vi "Text control 2 v5.4.vi"() -> ()   [LabVIEW 2016]
panel:
  in  "Tab Control":enum32{"Main", "Other parameters"}(tab)
  out "Line running":i32
  out "Total lines":i32
  out "Path":path=path "C:/users/rlp38/09Apr2009LTtesting/test2.txt"
  out "I vs Vg":cluster{"Y data in":dbl[], "X data in":dbl[]}[](graph)
  out "Is max":dbl format="%.2e"
  out "Id max":dbl format="%.2e"
  out "Ig max":dbl format="%.2e"
  out "Imax vs time":cluster{"Y data in":dbl[], "X data in":dbl[]}[](graph)
  out "Imin vs time":cluster{"Y data in":dbl[], "X data in":dbl[]}[](graph)
  out "I vs Vd":cluster{"Y data in":dbl[], "X data in":dbl[]}[](graph)
  in  "Script":string="#pulsedstressV d 0.03 20 0 0.5 0.0827 5\n#\n#itime m\n#gaterangemode a\n#drainrangemode a\n#pulsed on 0.05 0 0.02\n#transfer d -10 40 1 5 40 35\n#transfer d -10 40 1 5 40 35\n#transfer d -10 40 1 5 40 35\n#output d 0 40 20 0 40 1\n#\n#\n#sample 1 0.008 221 6 0.003\n#samplei 400e-6 200 6 0.002 0.1\n#vsu2pulse -10 4\n#\n#stressV 0.016 0.03 2e-4 0.1e-3 11\n#stressI 220e-7 0.08 15\n#transfer s -1 1 0.5 -0.005 0.005 0.005\n#output s 0 0 0 -0.008 0.008 0.002"
  out "Command running:":string
  out "Serial port data":string
  out "Elapsed Time":dbl caption="Elapsed Time (s)"
  in  "Units":u16(ring)=1 items=["Seconds", "Minutes", "Hours"]
  in  "Time Offset":dbl caption="Set Start Time (s)"
  in  "Reset":bool
  in  "Auto Reset":bool
  in  "integration time":u32(slide) max=2 step=1 scale=0.0..2.0
  in  "Interrupt run":bool
  out "Is on":dbl format="%.2e"
  out "Id on":dbl format="%.2e"
  out "Ig on":dbl format="%.2e"
  out "Ion vs time":cluster{"Y data in":dbl[], "X data in":dbl[]}[](graph)
  out "Ioff vs time":cluster{"Y data in":dbl[], "X data in":dbl[]}[](graph)
  out "Ig min":dbl format="%.2e"
  out "Id min":dbl format="%.2e"
  out "Is min":dbl format="%.2e"
  out "Is off":dbl format="%.2e"
  out "Id off":dbl format="%.2e"
  out "Ig off":dbl format="%.2e"
  in  "Step delay /s":dbl format="%.2f"
  in  "Integration time (long)":dbl=0.32 min=0.04 max=2.0 step=0.02 format="%.2f"
  in  "Integration time (short)":dbl=0.0019 min=8e-05 max=0.0019 step=8e-05 format="%^.0e"
  in  "delay time /s":dbl format="%.2f"
  in  "hold time /s":dbl format="%.2f"
  in  "Gate: Compliance":dbl=0.001 format="%.8f"
  in  "Drain: Compliance":dbl=0.001 format="%.8f"
  in  "Source/Drain Range":u8(slide)=6 max=11 scale=0.0..11.0
  in  "Source/Drain\nRange mode":u16(ring) items=["Auto", "Limited", "Fixed"]
  in  "Gate Range":u8(slide)=6 max=11 scale=0.0..11.0
  in  "Gate Range\nmode":u16(ring) items=["Auto", "Limited", "Fixed"]
  in  "Panel Controls":T1={"Emergency Stop"=refnum, "TransGraph Max"=1e-05, "Text/Graph (text=false)"=TRUE} {"TransGraph Max" format="%.2e"}
  in  "Panel Controls 2":T2={"Emergency Stop"=refnum, "TransGraph Max"=1e-05, "Text/Graph (text=false)"=TRUE, "TransGraph Min"=1e-11} {"TransGraph Min" format="%.2e"; "TransGraph Max" format="%.2e"}
  in  "SMU4":cluster{"on/off":bool, "Voltage":dbl} {"Voltage" min=-100.0 max=100.0 format="%.2f"}
  in  "Full Reset":bool
  in  "Standby":T3
  out "error out":errorcluster
  in  "Delay before read (ms)":u32=1000
  in  "byte count":u32=64
  in  "Serial End Mode for Reads":u16(ring)=2 items=["None", "LastBit", "TermChar"]
  in  "Timeout (ms)":u32=10000
  in  "Enable Termination\nChar (T)":bool=TRUE
  in  "Termination char\n(0xA = '\\n' = LF)\n(0xD = '\\r' = CR)":u8=13 format="%.0x"
  in  "flow control":u16(ring) items=["None"=0, "XON/XOFF"=1, "RTS/CTS"=2, "DTR/DSR"=4]
  in  "stop bits":u16(ring)=10 items=["1.0"=10, "1.5"=15, "2.0"=20]
  in  "parity":u16(ring) items=["None", "Odd", "Even", "Mark", "Space"]
  in  "data bits":u16=8 min=5 max=8 step=1
  in  "VISA resource name":refnum<visa-resource-name>="COM6"
  in  "baud rate":u32=9600
  in  "Gate":T4={"Gate Start"=0.0, "Gate Stop"=2.0, "Gate Step (linear only)"=1.0, "Gate Compliance"=0.0001, "Gate PComp"=0.0, "Range mode"=0, "Range"=6} {"Range" max=11 scale=0.0..11.0; "Range mode" items=["Auto", "Limited", "Fixed"]; "Gate PComp" format="%^.2e"; "Gate Compliance" format="%^.2e"; "Gate Step (linear only)" format="%^.4e"; "Gate Stop" format="%^.4e"; "Gate Start" format="%^.4e"}
  in  "Drain 2":T5={"Drain Start"=0.0, "Drain Stop"=2.0, "Drain Compliance"=0.0001, "Drain Step"=1.0, "Drain PComp"=0.0, "Range mode"=0, "Range"=6} {"Range" max=11 scale=0.0..11.0; "Range mode" items=["Auto", "Limited", "Fixed"]; "Drain PComp" format="%^.2e"; "Drain Step" format="%^.4e"; "Drain Compliance" format="%^.2e"; "Drain Stop" format="%^.4e"; "Drain Start" format="%^.4e"}
  in  "Timings 2":T6={"integration time"=0, "Short/Long integration time"=0.00064, "hold time (sec)"=0.0, "delay time (sec)"=0.0, "Step Time (0 disables)"=0.0, "sweep method"=0, "Pulse period"=0.005, "Base voltage"=0.0, "Pulse width"=0.0005} {"Pulse width" min=0.0005 max=0.1 step=0.0001 format="%.4f"; "Base voltage" format="%^.4e"; "Pulse period" min=0.005 max=1.0 step=0.0001 format="%.4f"; "sweep method" items=["Continuous", "Pulsed"]; "Step Time (0 disables)" format="%.2f"; "delay time (sec)" format="%.4f"; "hold time (sec)" format="%.4f"; "Short/Long integration time" format="%^.0e"; "integration time" scale=0.0..2.0}
  # "Time"
  # "1\n2\n3\n4\n5\n6\n7\n8\n9\n10\n11\n12\n13\n14\n15\n16\n17\n18\n19\n20"
  # "Syntax:\nitime [s|m|l]\ngaterangemode [a|l|f]\ndrainrangemode [a|l|f]\npulsed [on|off] PulsePeriod(sec) PulseBaseVoltage PulseONWidth(sec)\nstandby [on l off]\nwait NumMilliseconds\nwait-min NumMinutes\n# texthere = comment\ntransfer [s|d] VgStart VgStop VgStep VdStart VdStop VdStep\noutput [s|d] VgStart VgStop VgStep VdStart VdStop VdStep\nsample Vg Vd NumSamples Time(s) SampleInterval(s)\nsamplei Idg NumSamples Time(s) SampleInterval(s) VDGcompliance\n100 samples is approximately 13 seconds with medium integration\n# if in doubt use SampleInterval(s) = 0.004\nstressV VG VD IGcompliance IDcompliance Duration(sec)\nstressI IDG VDGcompliance Duration(sec)\nvsu2pulse Bias Duration(s)\npulsedstressV [s|d] VEstop VgON VgOFF Period(s) PulseONwidth(s) Vd\nsample-fpp Vg Vd NumSamples Time\nresample-fpp Vg Vd\ntransfer-fpp [s|d] VgStart VgStop VgStep VdStart VdStop VdStep\noutput-fpp [s|d] VgStart VgStop VgStep VdStart VdStop VdStep\nserial SerialPortCommand"
  # "Serial port settings"
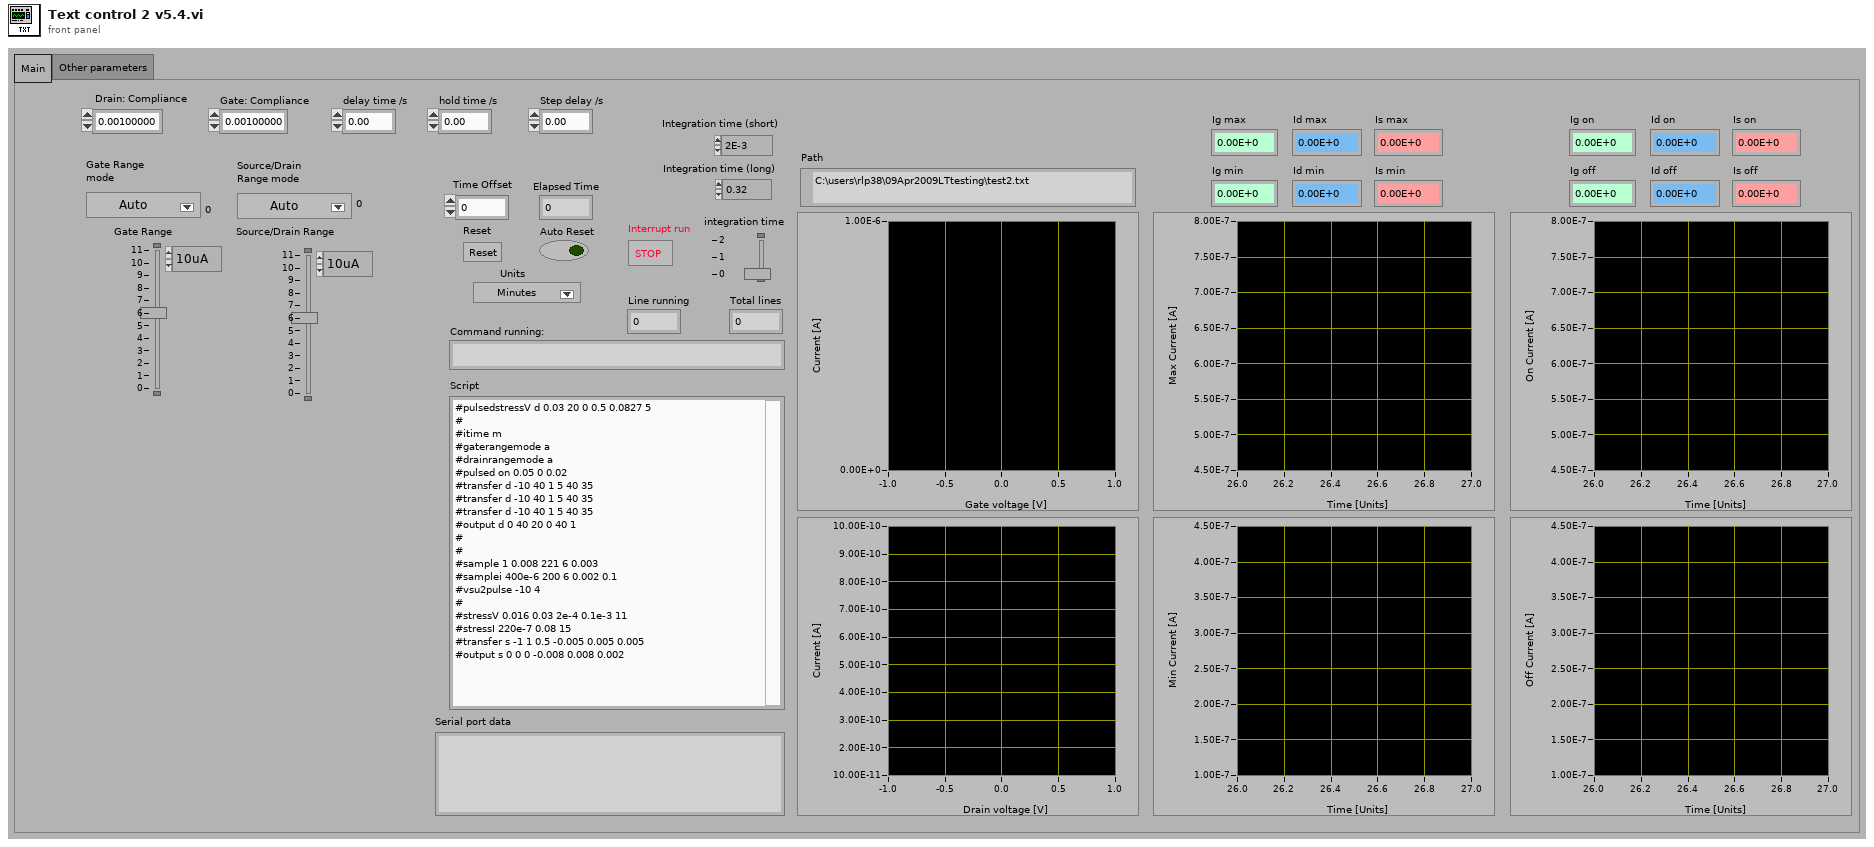
[diagram p1: front panel]
types:
  T1 = cluster{"Emergency Stop":refnum<vi>, "TransGraph Max":dbl, "Text/Graph (text=false)":bool}
  T2 = cluster{"Emergency Stop":refnum<vi>, "TransGraph Max":dbl, "Text/Graph (text=false)":bool, "TransGraph Min":dbl}
  T3 = cluster{"Gate Standby":bool, "Drain Standby":bool}
  T4 = cluster{"Gate Start":dbl, "Gate Stop":dbl, "Gate Step (linear only)":dbl, "Gate Compliance":dbl, "Gate PComp":dbl, "Range mode":u16, "Range":u8}
  T5 = cluster{"Drain Start":dbl, "Drain Stop":dbl, "Drain Compliance":dbl, "Drain Step":dbl, "Drain PComp":dbl, "Range mode":u16, "Range":u8}
  T6 = cluster{"integration time":u32, "Short/Long integration time":dbl, "hold time (sec)":dbl, "delay time (sec)":dbl, "Step Time (0 disables)":dbl, "sweep method":u16, "Pulse period":dbl, "Base voltage":dbl, "Pulse width":dbl}
  T7 = enum16{"open", "replace", "create", "open or create", "replace or create", "replace or create with confirmation"}
  T8 = cluster{"V2 Start":dbl, "V2 Step":dbl, "Number of points":i32}
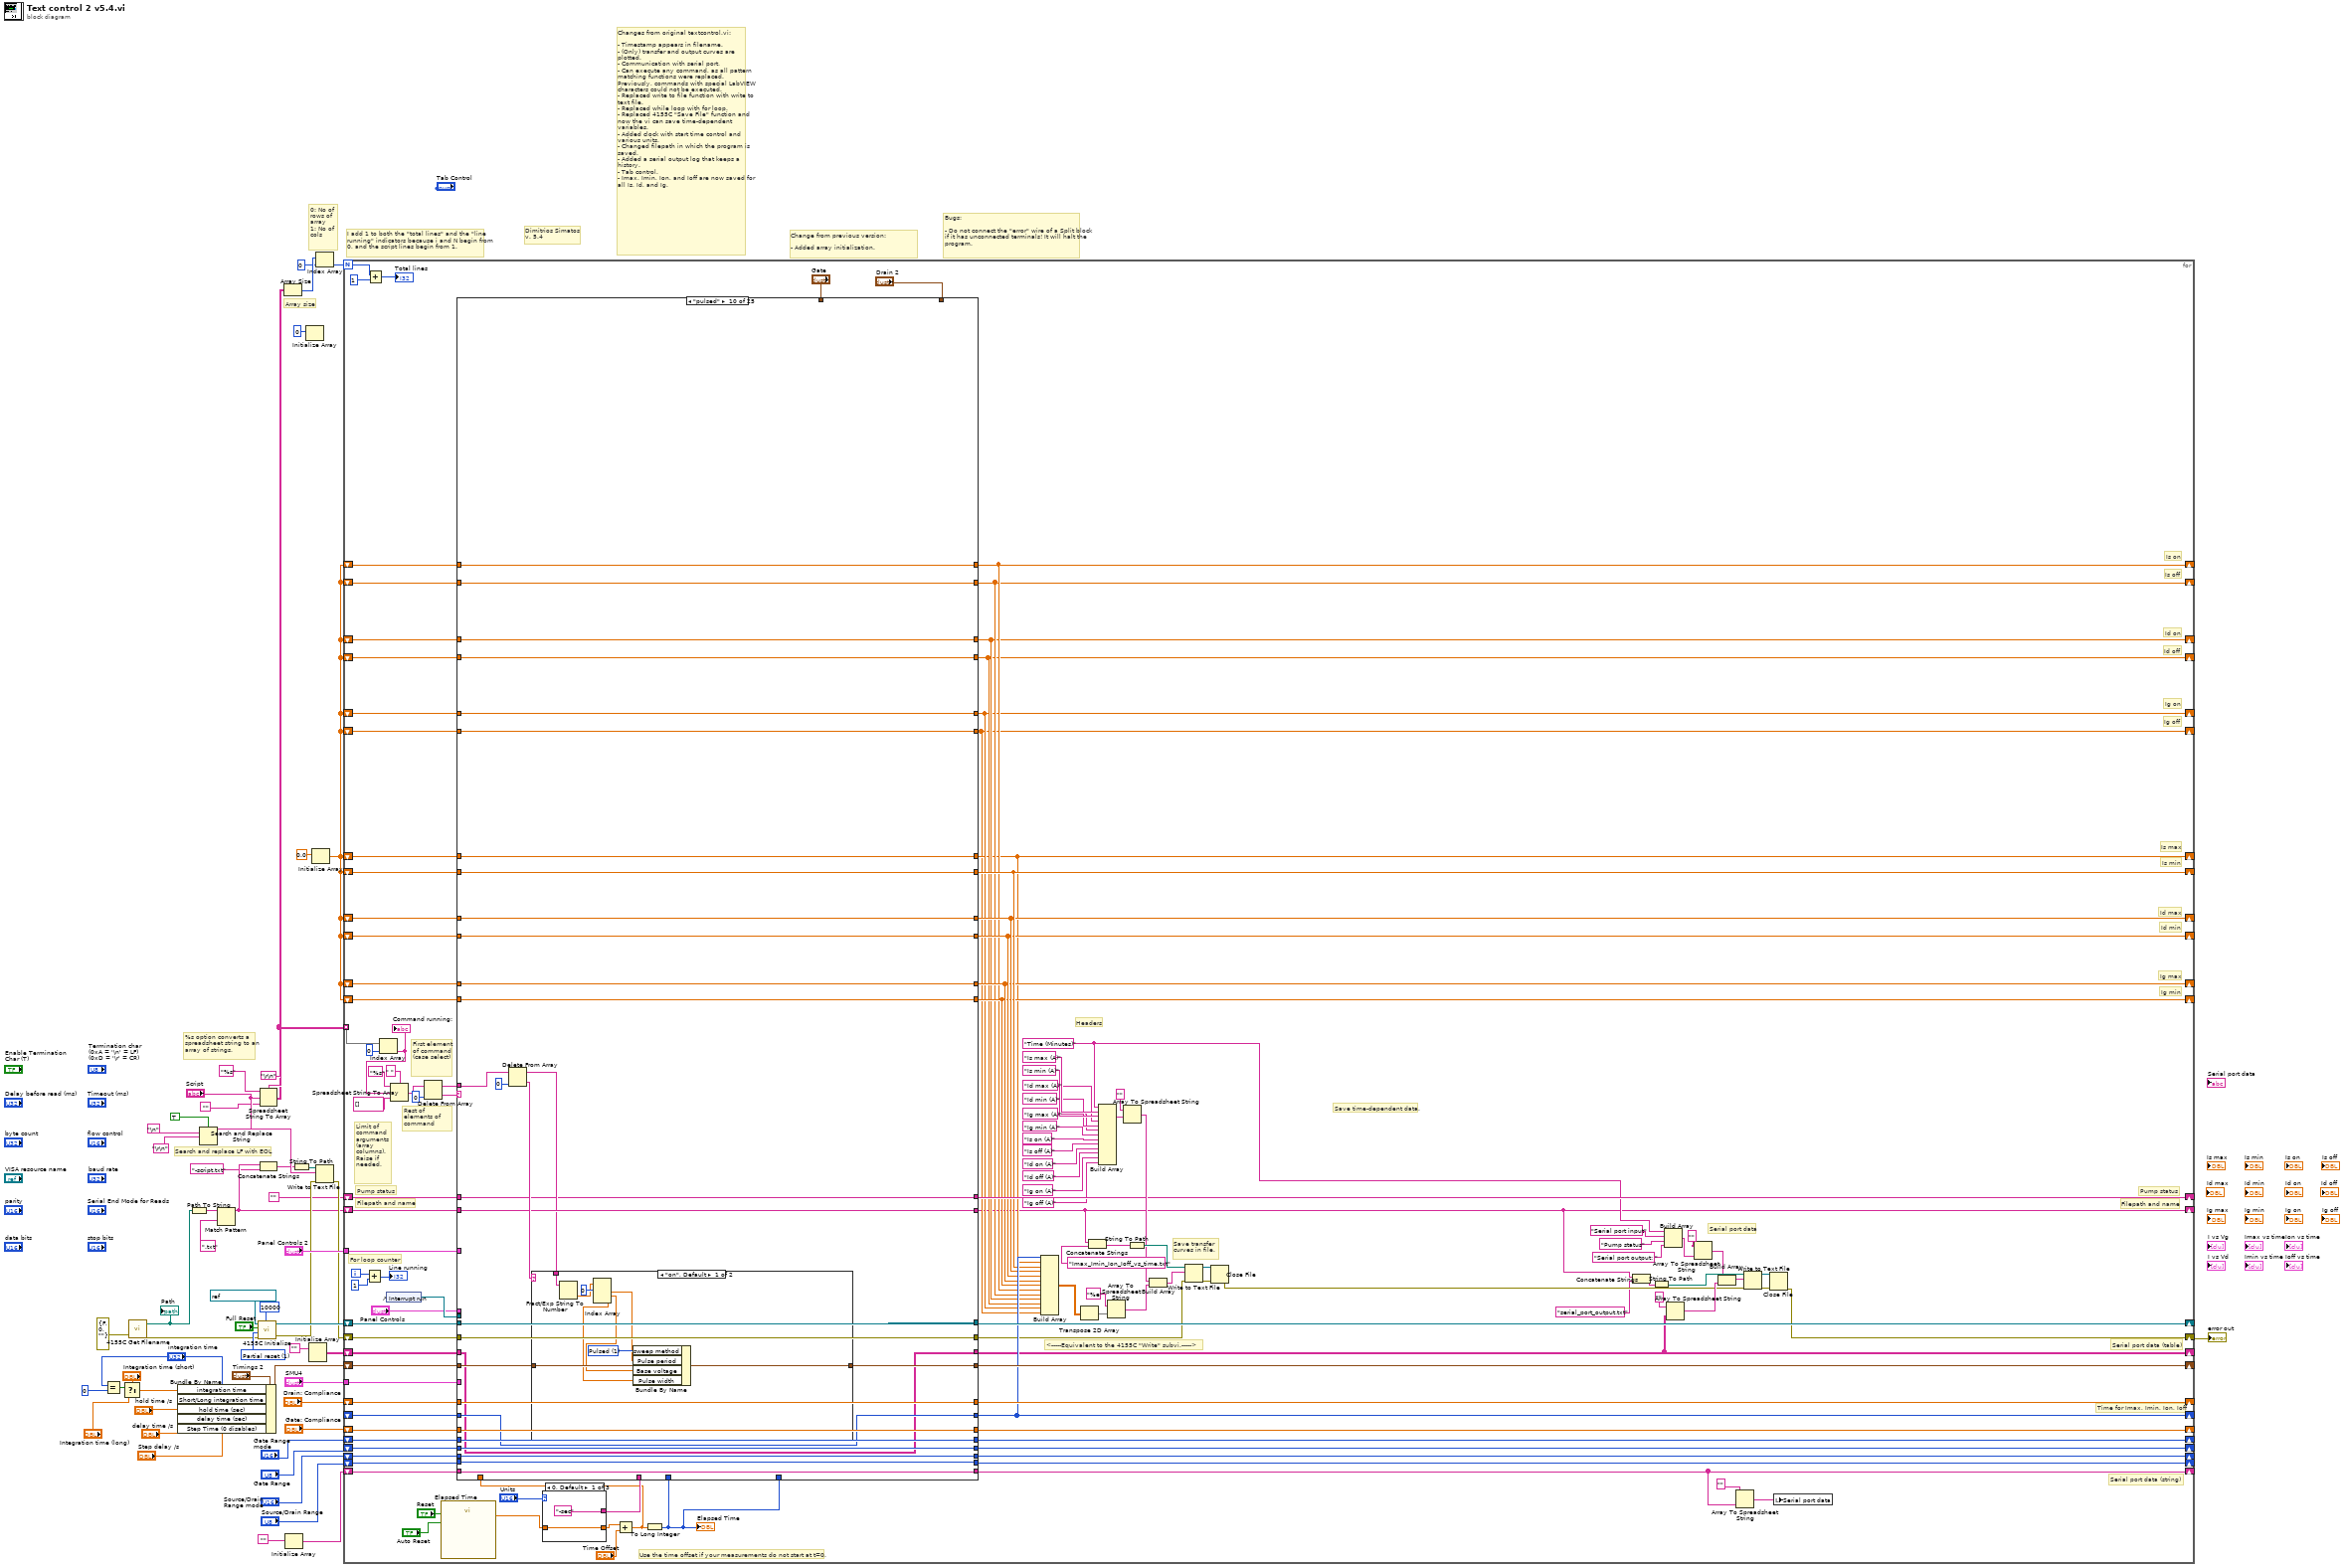
[diagram p0: block diagram]
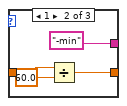
[diagram p2: hidden frame]
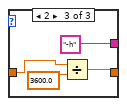
[diagram p3: hidden frame]
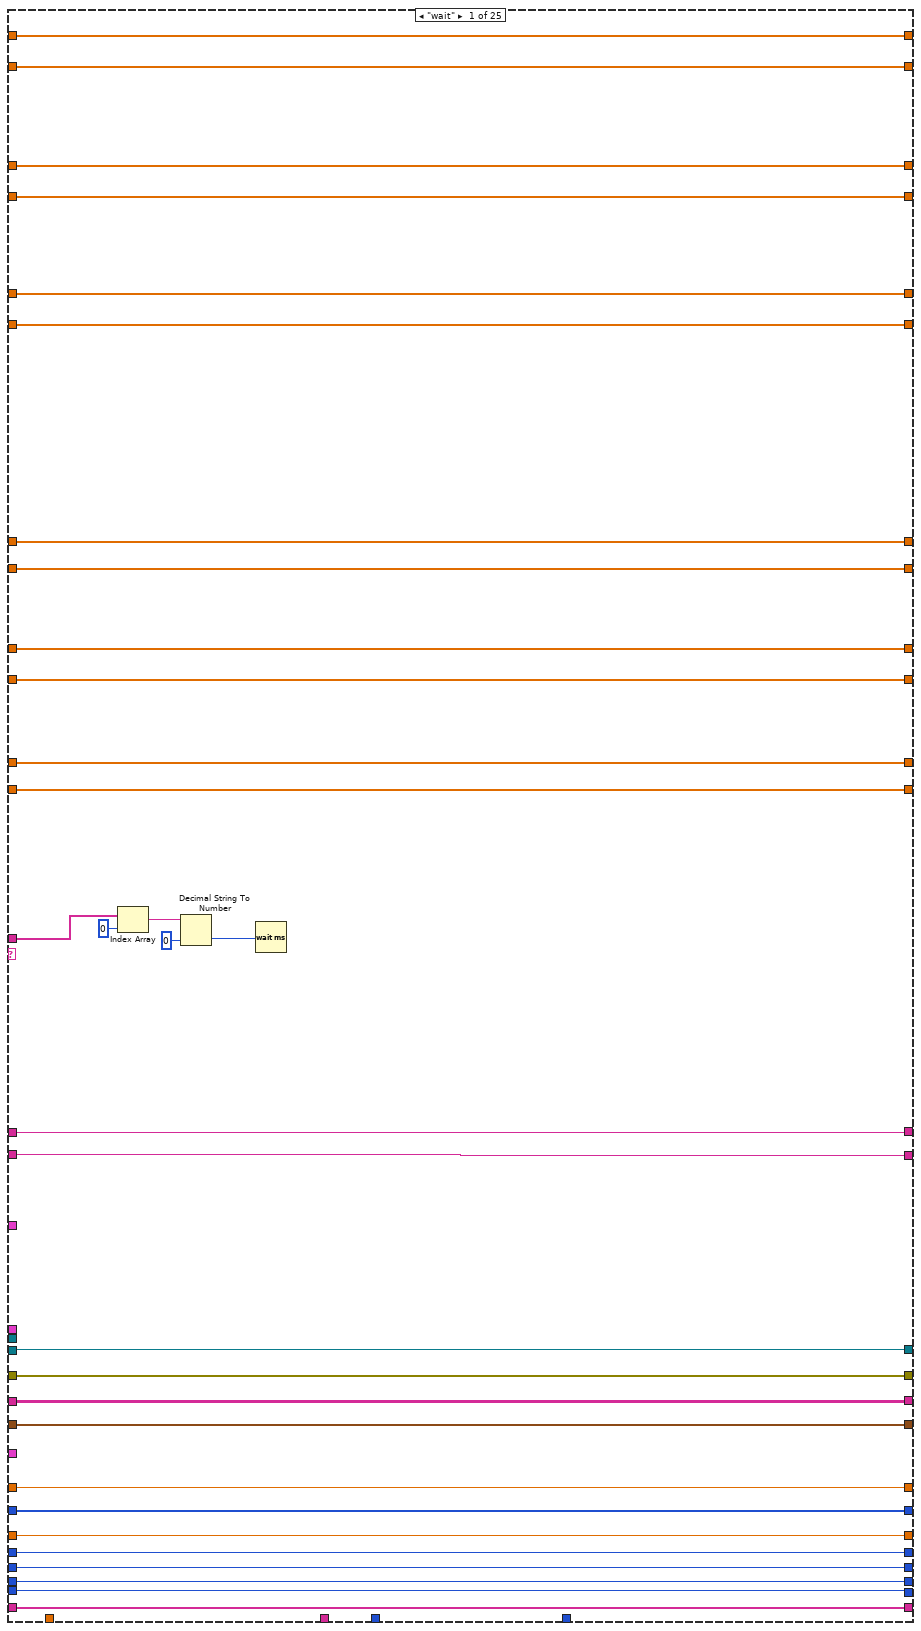
[diagram p4: hidden frame]
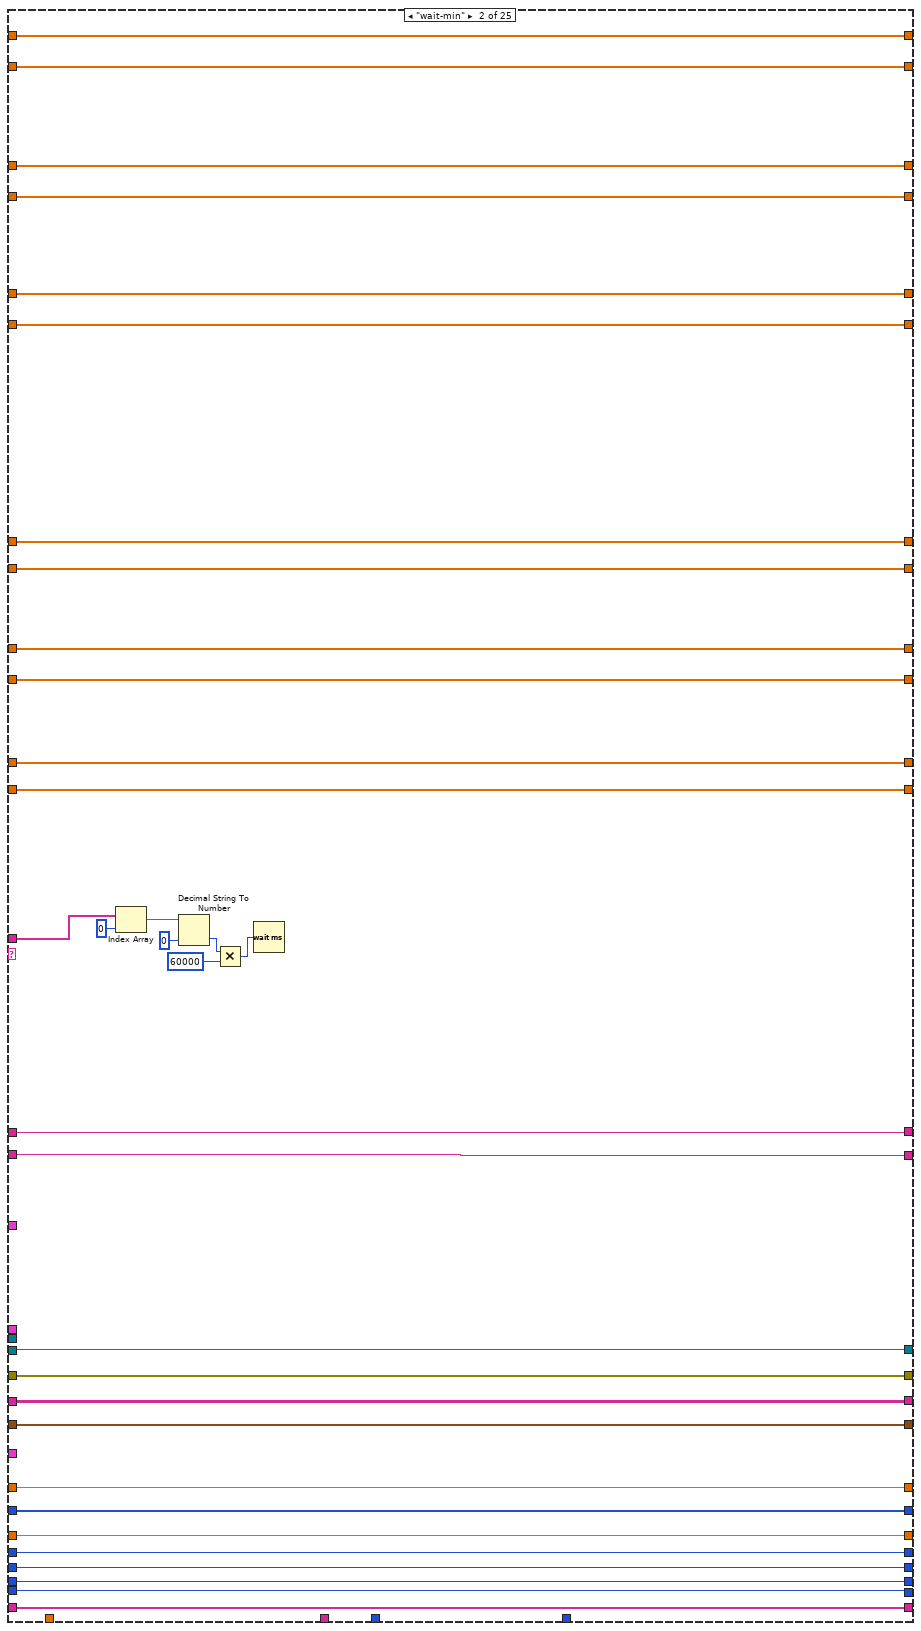
[diagram p5: hidden frame]
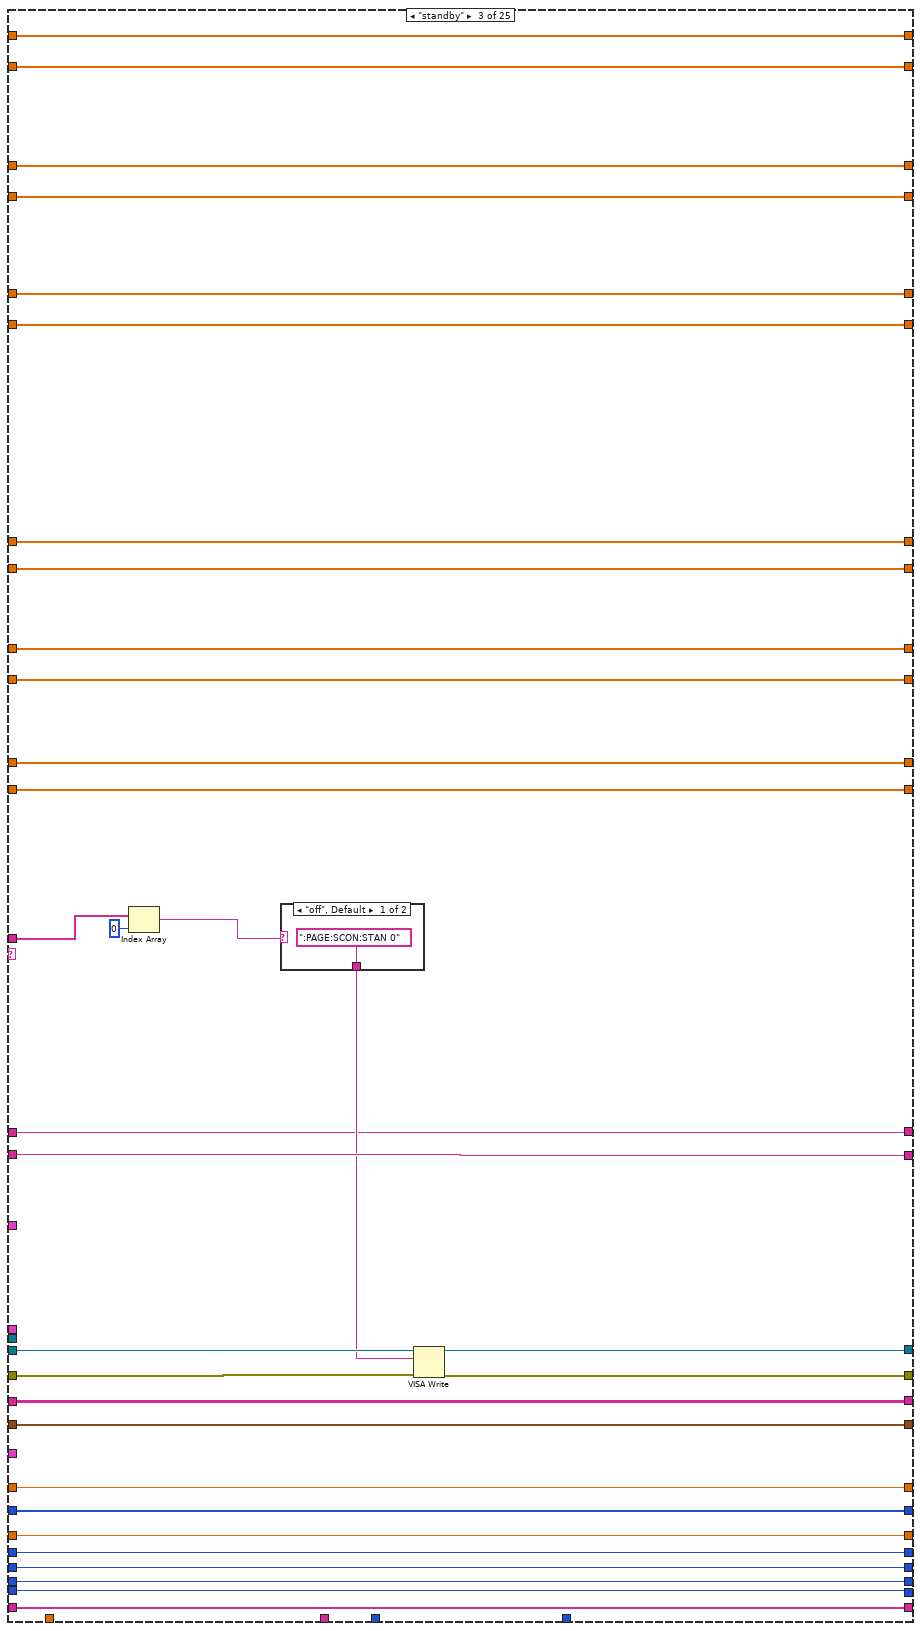
[diagram p6: hidden frame]
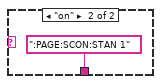
[diagram p7: hidden frame]
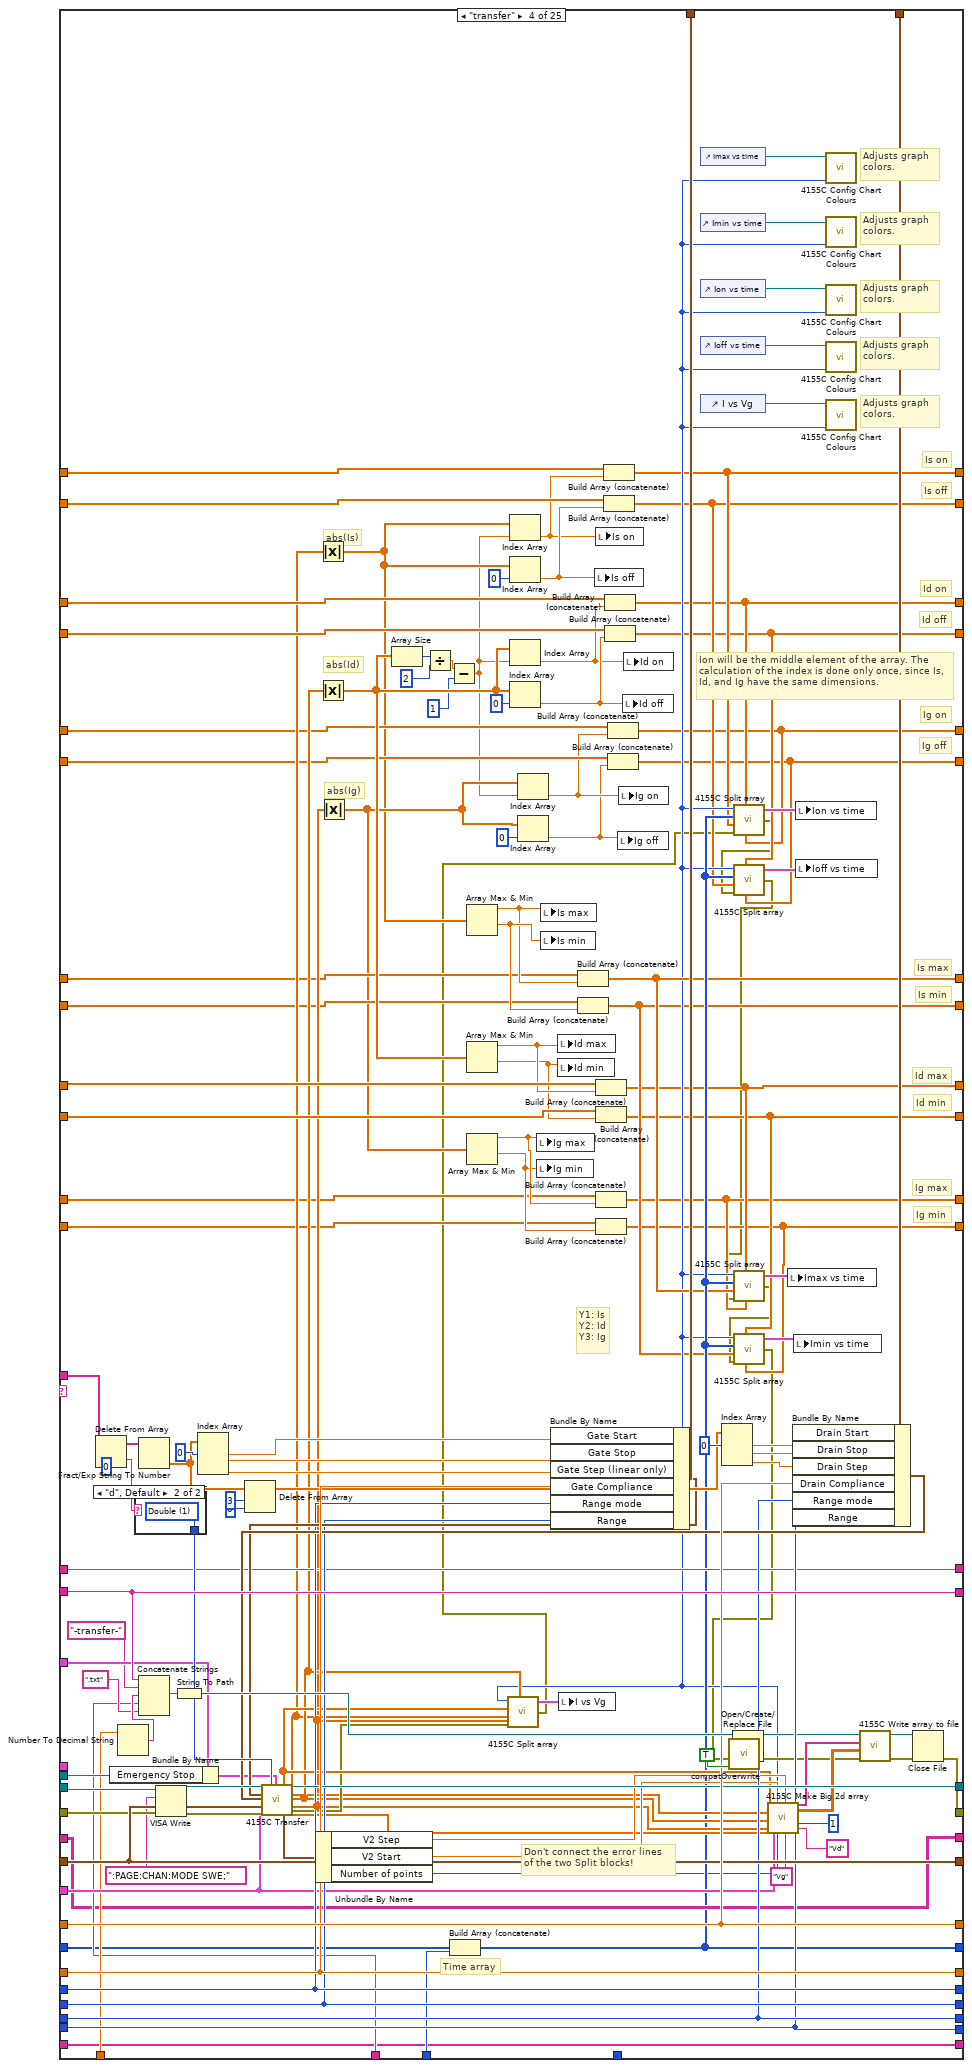
[diagram p8: hidden frame]
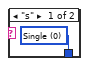
[diagram p9: hidden frame]
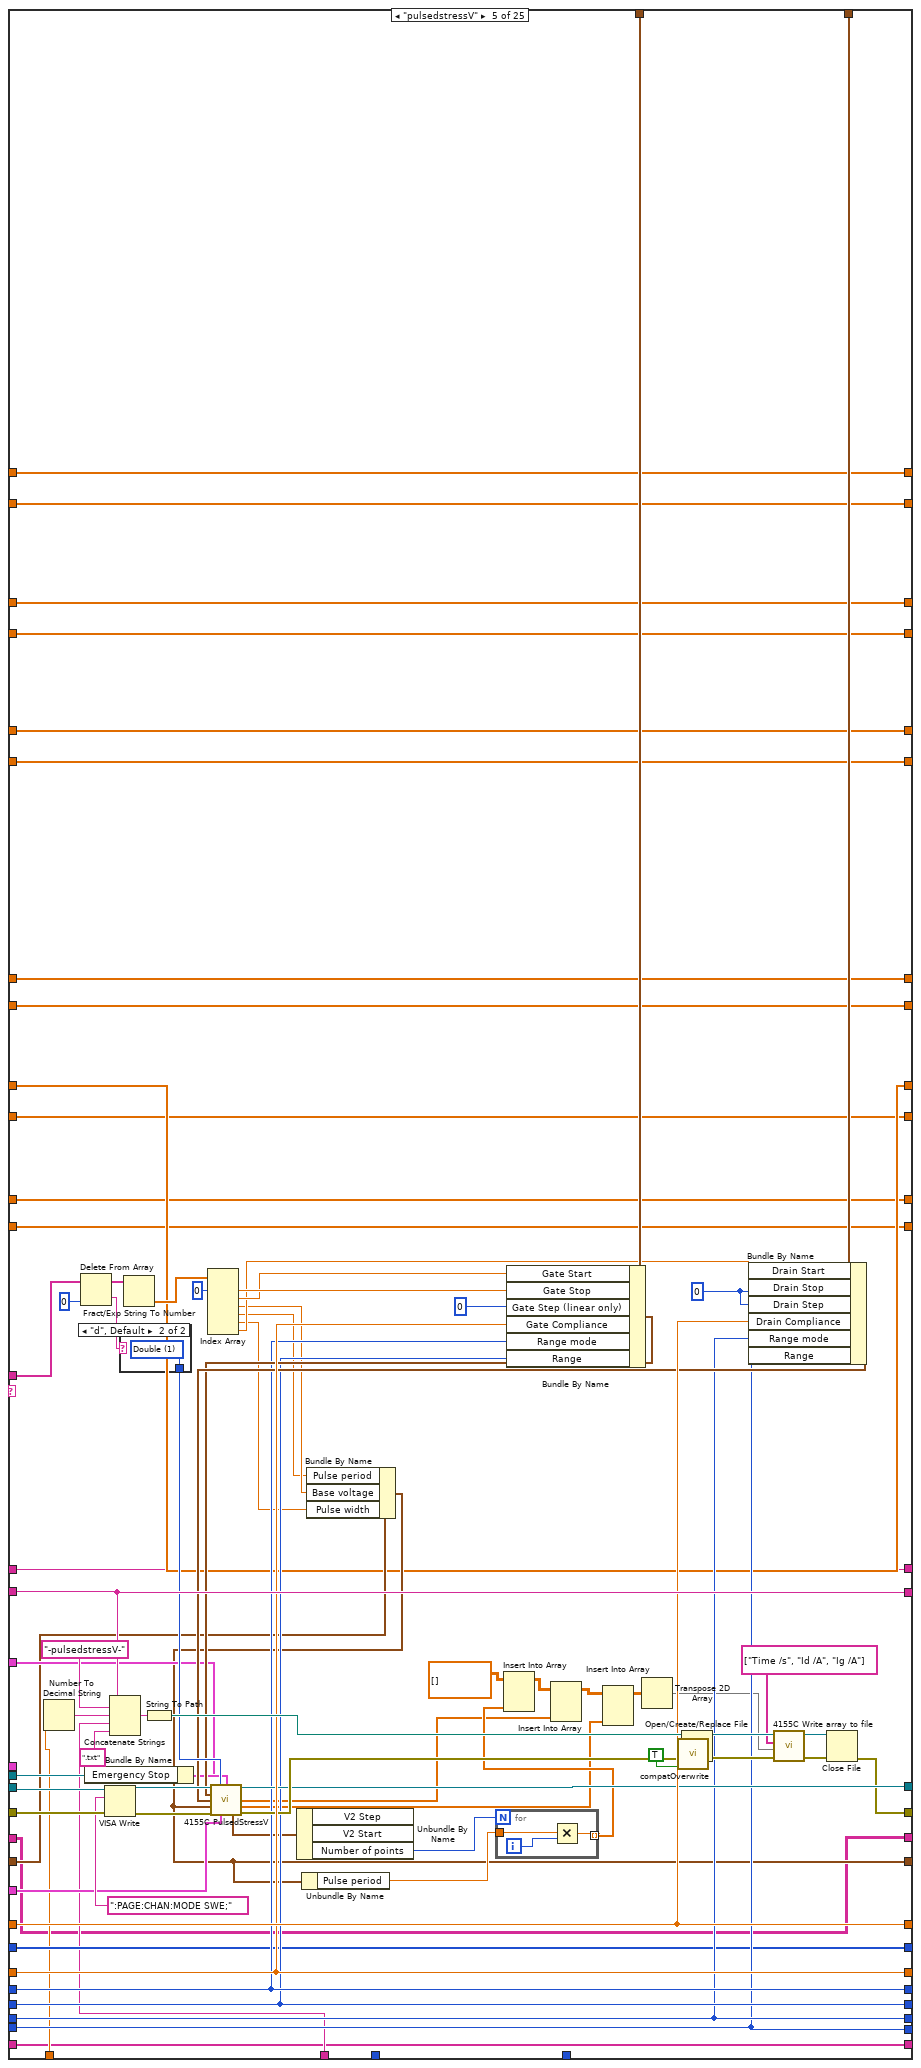
[diagram p10: hidden frame]
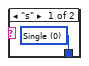
[diagram p11: hidden frame]
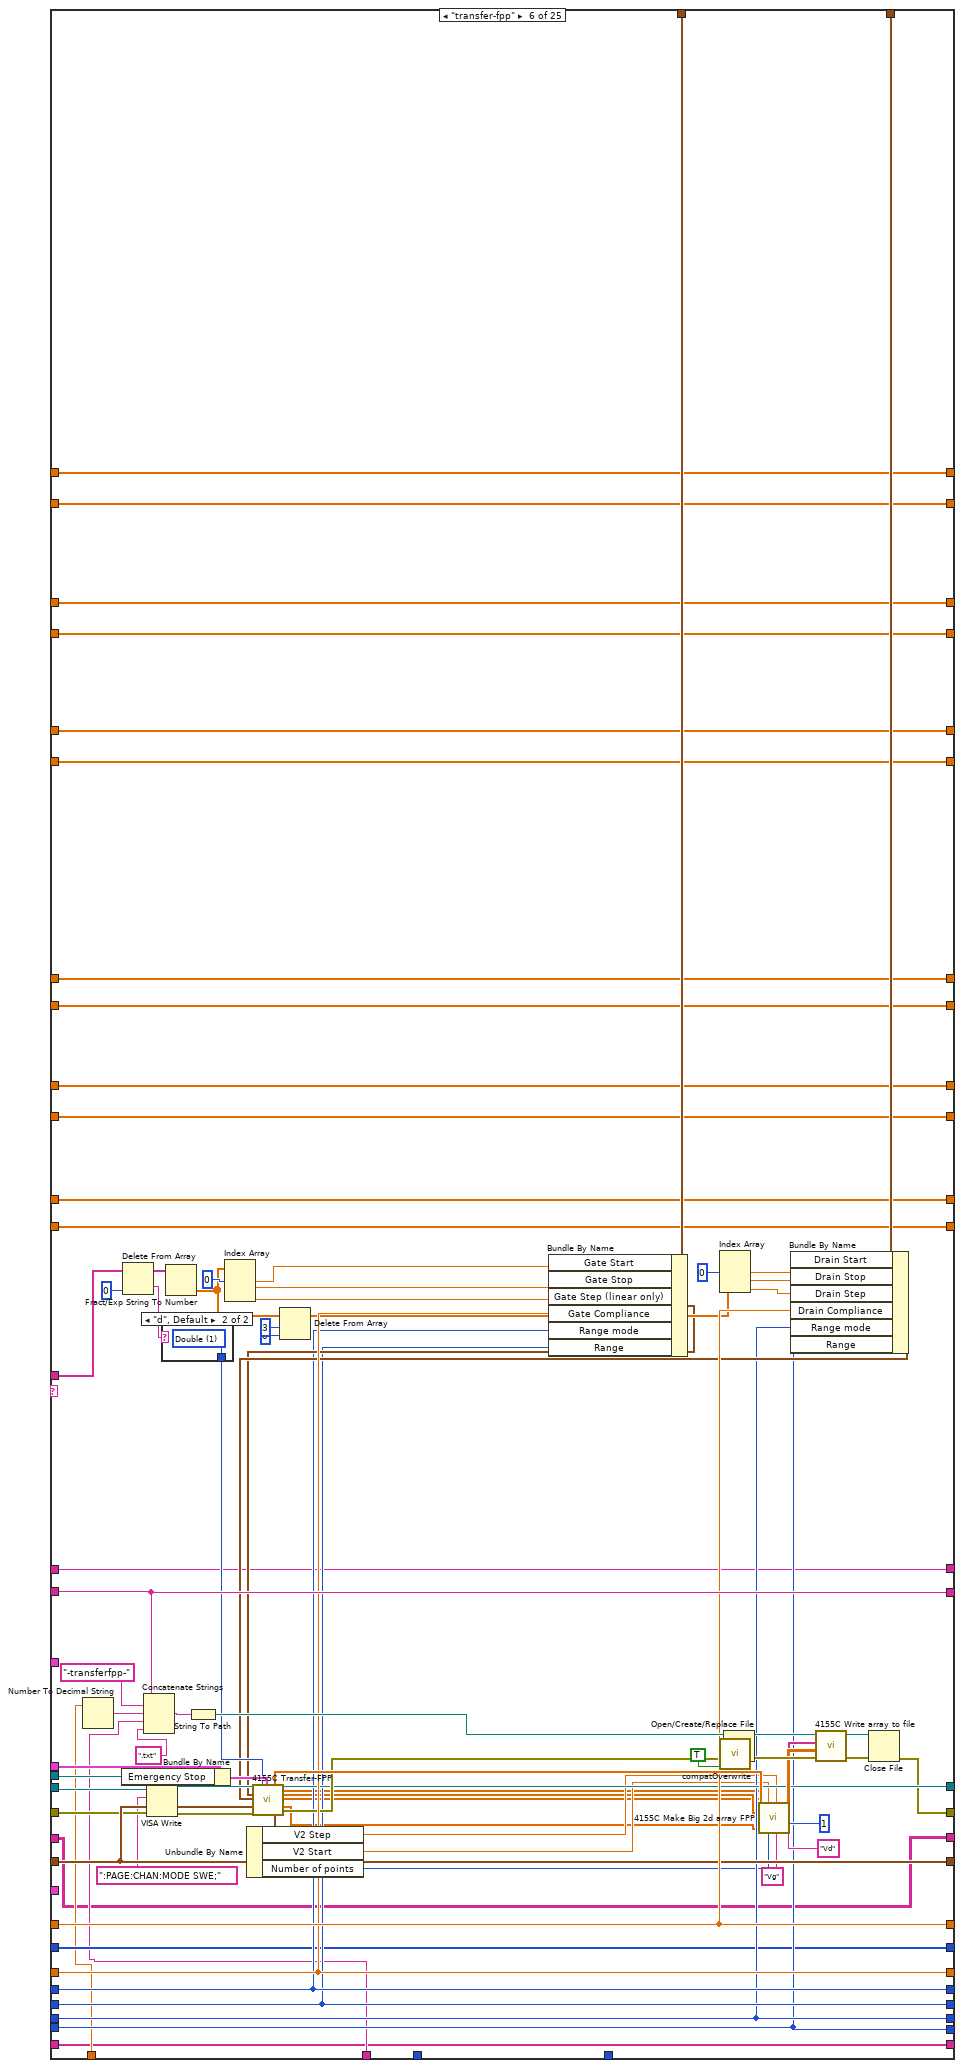
[diagram p12: hidden frame]
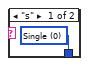
[diagram p13: hidden frame]
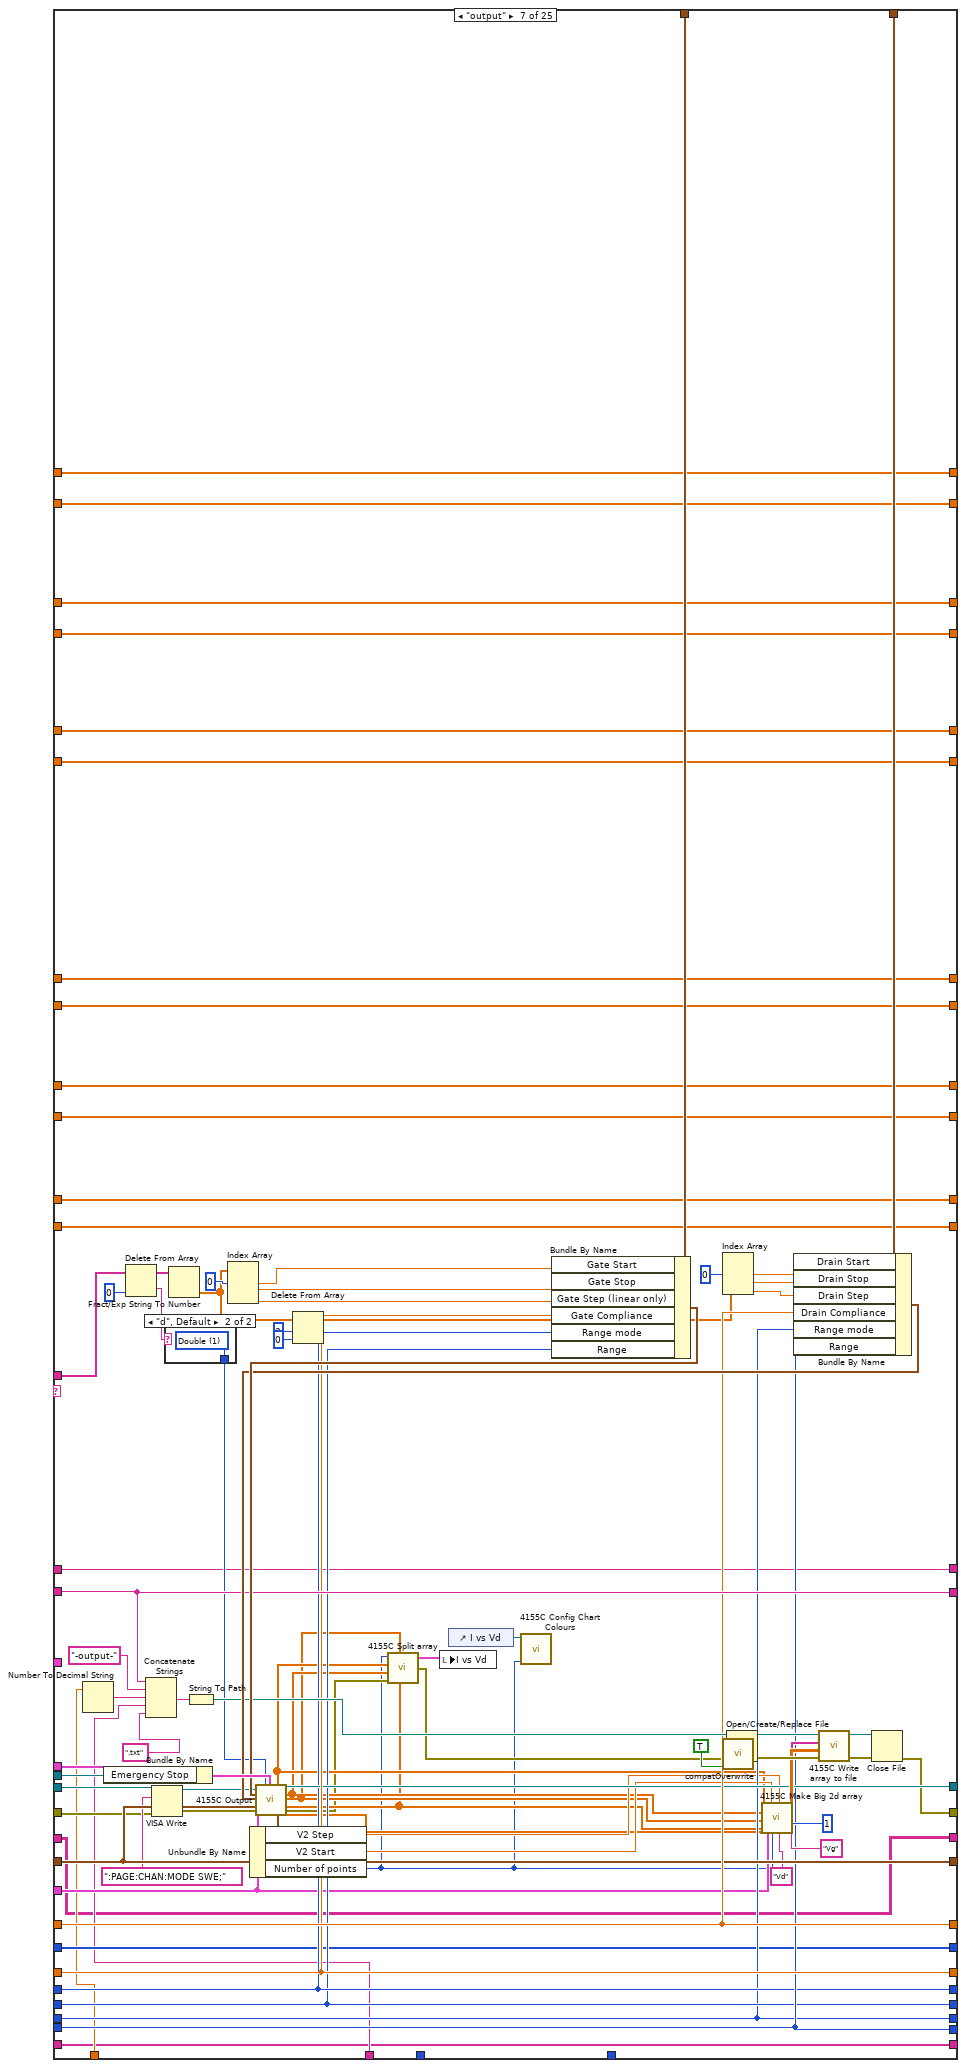
[diagram p14: hidden frame]
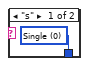
[diagram p15: hidden frame]
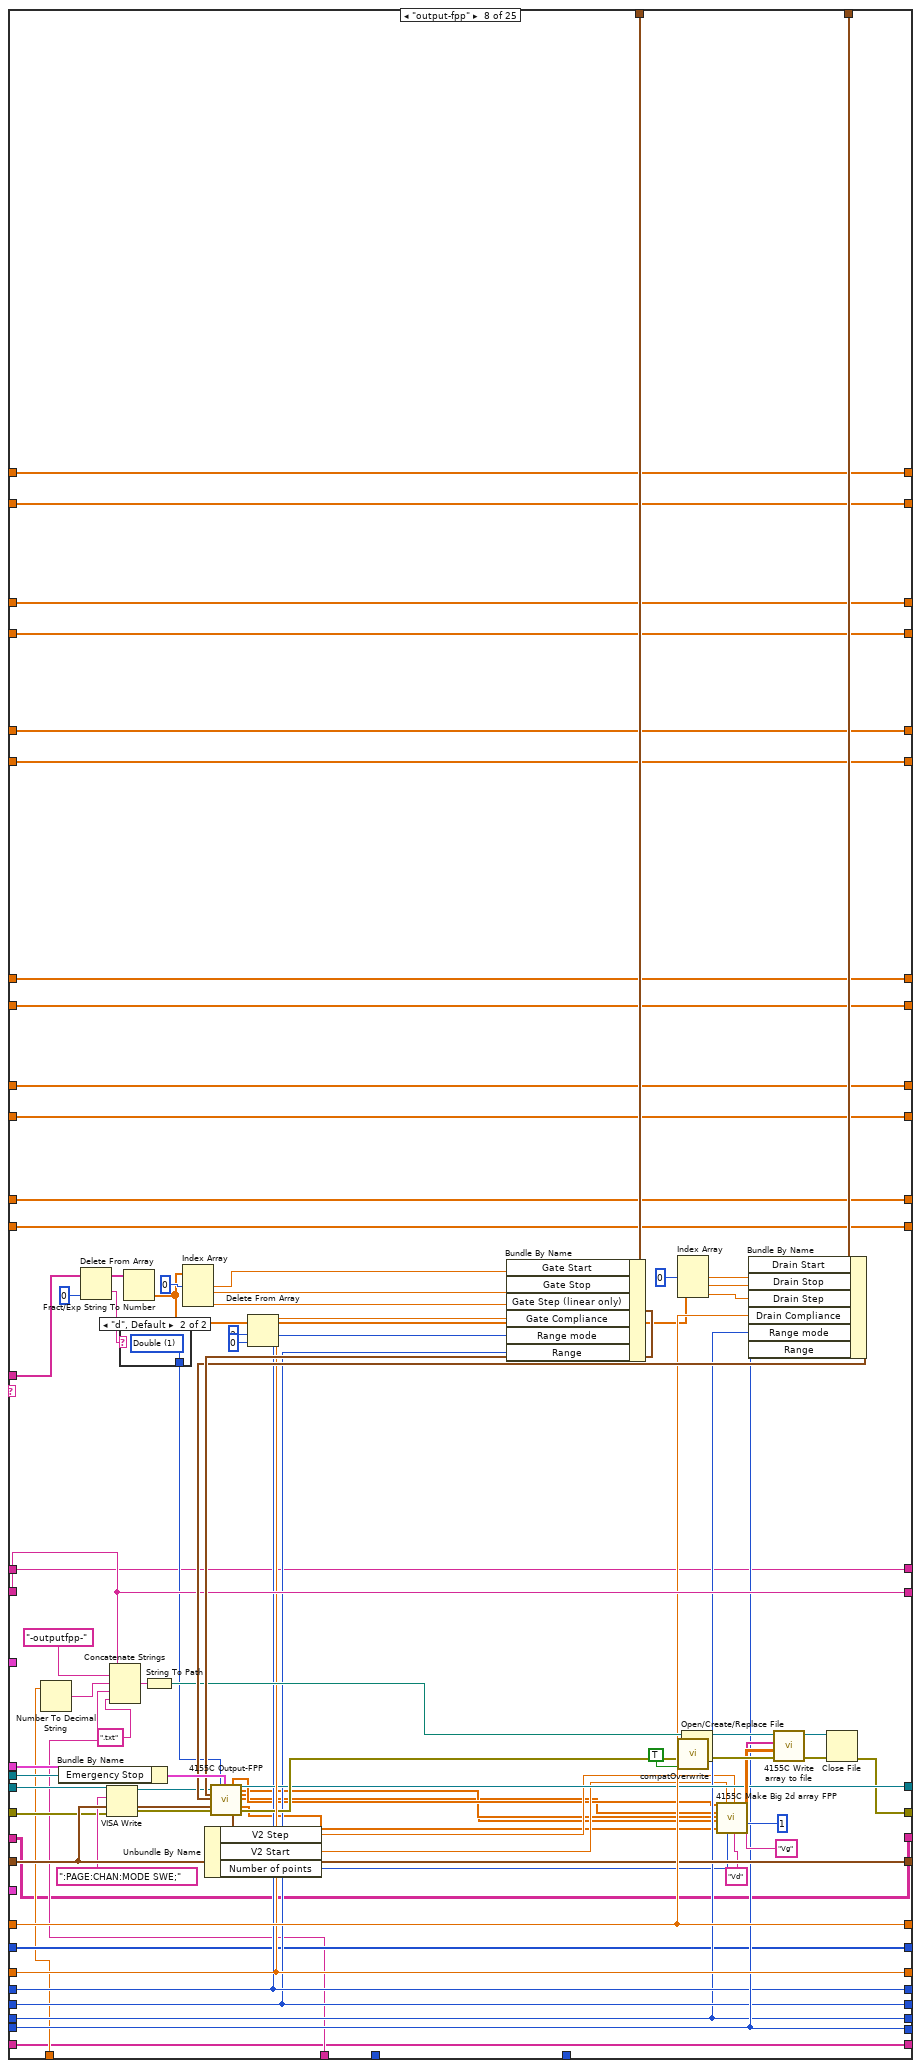
[diagram p16: hidden frame]
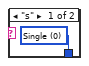
[diagram p17: hidden frame]
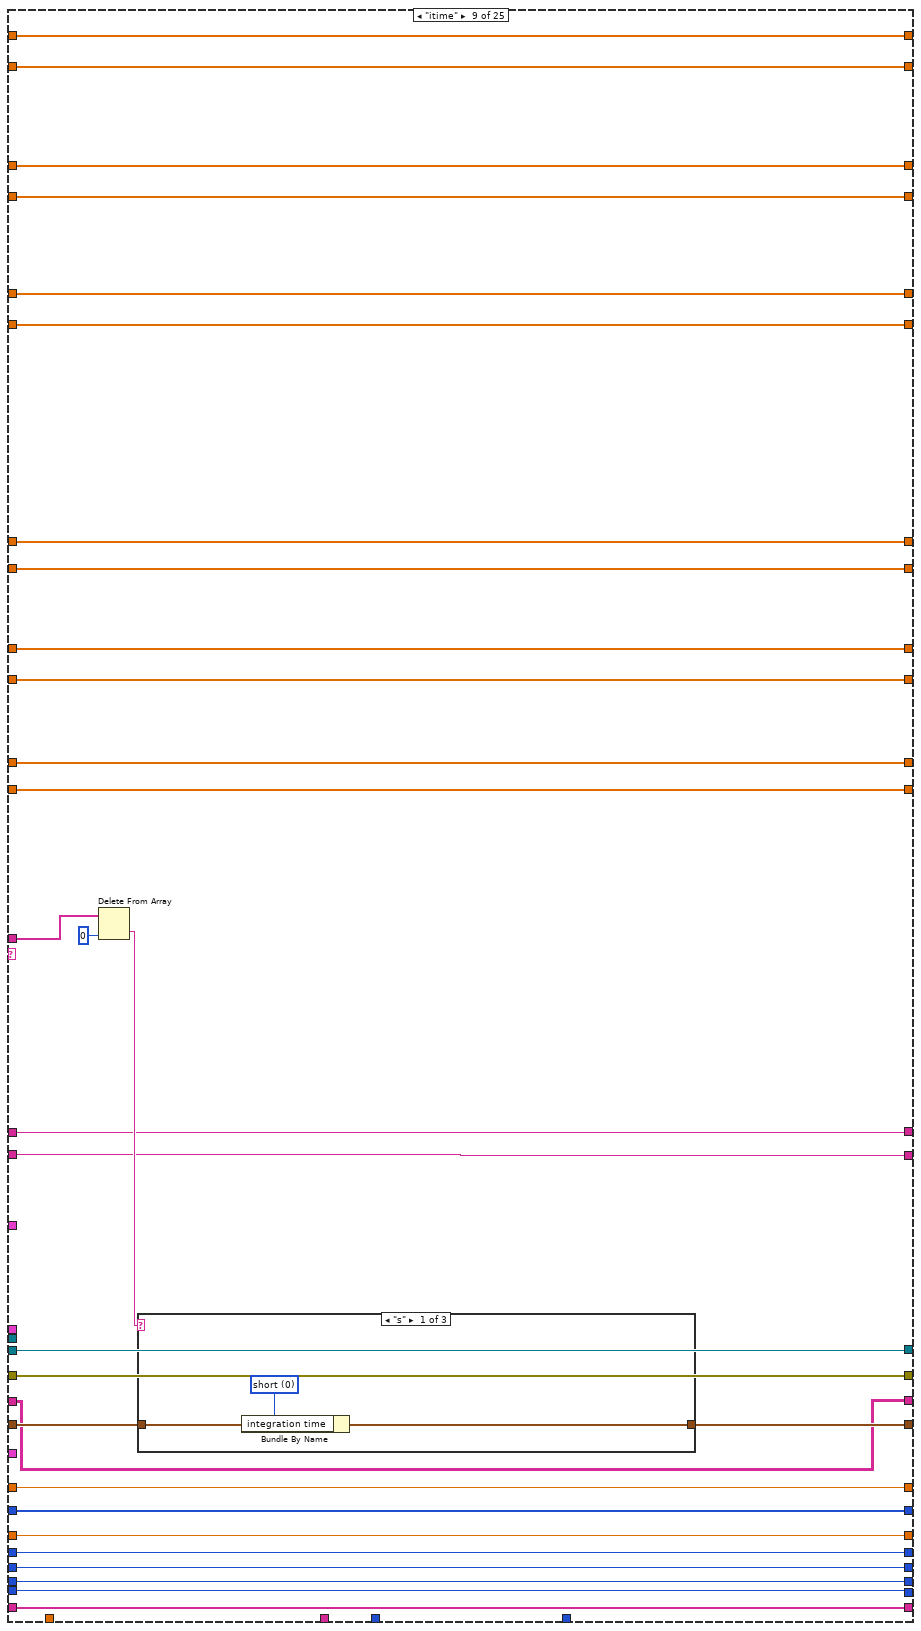
[diagram p18: hidden frame]
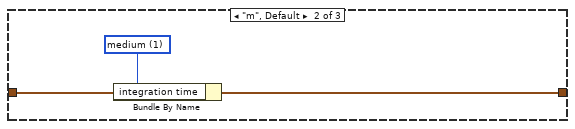
[diagram p19: hidden frame]
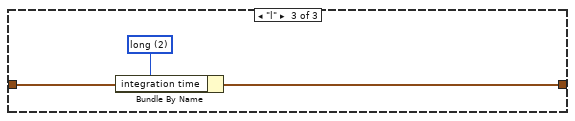
[diagram p20: hidden frame]
diagram:
  w47 = u16 1 items=["Reset All", "Partial reset"] ("Type of reset")
  # "Change from previous version:\n\n- Added array initialization."
  # "I add 1 to both the \"total lines\" and the \"line running\" indicators because i and N begin from 0, and the script lines begin from 1."
  # "Bugs:\n\n- Do not connect the \"error\" wire of a Split block if it has unconnected terminals! It will halt the program."
  # "Array size"
  # "%s option converts a spreadsheet string to an array of strings."
  # "0: No of rows of array\n1: No of cols"
  # "Dimitrios Simatos\nv. 5.4"
  # "Changes from original textcontrol.vi:\n\n- Timestamp appears in filename.\n- (Only) transfer and output curves are plotted.\n- Communication with serial port.\n- Can execute any command, as all pattern matching functions were replaced. Previously, commands with special LabVIEW characters could not be executed.\n- Replaced write to file function with write to text file.\n- Replaced while loop with for loop.\n- Replaced 4155C \"Save File\" function and now the vi can save time-dependent variables.\n- Added clock with start time control and various units.\n- Changed filepath in which the program is saved.\n- Added a serial output log that keeps a history.\n- Tab control.\n- Imax, Imin, Ion, and Ioff are now saved for all Is, Id, and Ig."
  # "Search and replace LF with EOL"
  n1 = Equal?(x="integration time", y=u32 0) -> (x = y?=w51:bool)
  n2 = Select(t="Integration time (short)", s=w51, f="Integration time (long)") -> (s? t:f=w55:dbl)
  n3 = call "4155C Get Filename.vi"("error in (no error)"=errorcluster {"status"=FALSE, "code"=0, "source"=""}) -> ("error out"=w42:errorcluster, "path"=w17:path)  [unwired: 2 in, 1 out]
  "Path" <- w17
  n4 = Bundle By Name(cluster="Timings 2", "integration time"="integration time", "Short/Long integration time"=w55, "hold time (sec)"="hold time /s", "delay time (sec)"="delay time /s", "Step Time (0 disables)"="Step delay /s") -> (w40:T6)
  n5 = Path To String(path=w17) -> (string=w18:string)
  n6 = Search and Replace String(replace all?=TRUE ("replace all? (F)"), input string="Script", search string="\n", replace string="\r\n") -> (result string=w30:string)  [unwired: 4 in, 3 out]
  n7 = Match Pattern(string=w18, regular expression=".txt") -> (before substring=w2:string)  [unwired: 1 in, 3 out]
  n8 = call "4155C Initialise.vi"("VISA resource name in"=refnum<visa-resource-name> "GPIB0::14::INSTR", "Reset"="Full Reset", "Type of reset"=w47, "error in (no error)"=w42, "VISA Timeout Value"=u32 10000) -> ("VISA Resource Name out"=w41:refnum<visa-resource-name>, "error out"=w13:errorcluster)
  n9 = Spreadsheet String To Array(delimiter (Tab)="\r\n", format string="%s", spreadsheet string="Script", array type (2D Dbl)="") -> (array=w21:string[][])
  n10 = Concatenate Strings(w2, "-script.txt" ("regular expression")) -> (w3:string)
  n11 = Array Size(array=w21) -> (size(s)=w25:i32[])
  n12 = Initialize Array("") -> (w7:string[])  [unwired: 1 in]
  n13 = String To Path(string=w3) -> (path=w14:path)
  n14 = Initialize Array(0 ("element")) -> ()  [unwired: 1 in, 1 out]
  n15 = Initialize Array("") -> (w5:string[][])  [unwired: 2 in]
  n16 = Initialize Array(0.0 ("element")) -> (w10:dbl[])  [unwired: 1 in]
  n17 = Index Array(array=w25, index=0) -> (element=w23:i32)
  n18 = Write to Text File(file (use dialog)=w14, text=w30, error in=w13) -> (error out=w12:errorcluster)  [unwired: 1 in, 2 out]
  n19 = for {
    N: w23 -> [w125]
    tunnel: "SMU4" -> [w161]
    shift-left: "Source/Drain Range" -> [w166]
    shift-right: [w162] -> _
    shift-left: "Source/Drain\nRange mode" -> [w167]
    shift-right: [w163] -> _
    shift-left: "Gate Range" -> [w168]
    shift-right: [w164] -> _
    shift-left: "Gate Range\nmode" -> [w169]
    shift-right: [w165] -> _
    shift-left: "Gate: Compliance" -> [w178]
    shift-right: [w174] -> _
    shift-left: "Drain: Compliance" -> [w179]
    shift-right: [w175] -> _
    shift-left: w40 -> [w180]
    shift-right: [w176] -> _
    shift-left: w12 -> [w181]
    shift-right: [w59] -> w16
    shift-left: w41 -> [w182]
    shift-right: [w177] -> _
    shift-left: w2 -> [w183]
    shift-right: [w57] -> _
    tunnel: "Panel Controls 2" -> [w160]
    shift-right: [w72] -> _
    shift-left: w10 -> [w159]
    shift-right: [w110] -> _
    shift-left: _ -> [w155]
    tunnel: w21 -> [w154] mode=indexing
    shift-right: [w71] -> _
    shift-left: w10 -> [w131]
    shift-right: [w104] -> _
    shift-left: w7 -> [w117]
    shift-right: [w112] -> _
    shift-left: "" -> [w111]
    shift-right: [w105] -> _
    shift-left: w5 -> [w107]
    shift-right: [w65] -> _
    shift-left: w10 -> [w93]
    shift-right: [w66] -> _
    shift-left: w10 -> [w92]
    shift-right: [w70] -> _
    shift-left: w10 -> [w81]
    shift-right: [w69] -> _
    shift-left: w10 -> [w80]
    shift-right: [w63] -> _
    shift-left: w10 -> [w79]
    shift-right: [w73] -> _
    shift-left: w10 -> [w78]
    shift-right: [w64] -> _
    shift-left: w10 -> [w77]
    shift-right: [w62] -> _
    shift-left: w10 -> [w76]
    shift-right: [w68] -> _
    shift-left: w10 -> [w75]
    shift-right: [w67] -> _
    shift-left: w10 -> [w74]
    i -> [w120]
    w95 = "Time (Minutes)" ("element")
    # "Is off"
    # "Is on"
    # "Ig off"
    # "Ig on"
    # "Is min"
    # "Is max"
    # "Ig min"
    # "Ig max"
    # "Id min"
    # "Id max"
    # "Id off"
    # "Id on"
    # "Pump status"
    # "Filepath and name"
    # "Pump status"
    # "Limit of command arguments (array columns). Raise if needed."
    # "Serial port data (string)"
    # "Serial port data (table)"
    # "Serial port data"
    # "For loop counter"
    # "<-----Equivalent to the 4155C \"Write\" subvi.----->"
    # "Headers"
    # "Save transfer curves in file."
    # "Filepath and name"
    # "Save time-dependent data."
    # "Use the time offset if your measurements do not start at t=0."
    # "Time for Imax, Imin, Ion, Ioff"
    # "Rest of elements of command"
    # "First element of command\n(case select)"
    n20 = Add(x=w120, y=1) -> (x+y=→"Line running":i32)
    n21 = Add(x=w125, y=1) -> (x+y=→"Total lines":i32)
    n22 = Index Array(array=w154, index=0 ("line index")) -> (element=w149:string)
    "Command running:" <- w149
    n23 = control-ref of="Interrupt run"() -> (w173:refnum<vi>)
    n24 = Spreadsheet String To Array(delimiter (Tab)=" ", format string="%s", spreadsheet string=w149, array type (2D Dbl)=string[] []) -> (array=w147:string[])
    n25 = Delete From Array(array=w147, index=0) -> (deleted portion=w94:string, array with subset deleted=w146:string[])  [unwired: 1 in]
    n26 = call "Elapsed Time"("Reset"="Reset", "Auto Reset"="Auto Reset") -> ("Elapsed Time (s)"=w156:dbl)  [unwired: 10 in, 7 out]
    n27 = case shown="0, Default" "Units" {
      tunnel: ["-sec" "-min" "-h"] -> w157
      tunnel: [w184 w188 w191] -> w127
      tunnel: w156 -> [w184 w187 w192]
      frame 0, Default {
      }
      frame 1 {
        n28 = Divide(x=w187, y=60.0) -> (x/y=w188:dbl)
      }
      frame 2 {
        n29 = Divide(x=w192, y=3600.0) -> (x/y=w191:dbl)
      }
    }
    n30 = Add(x=w127, y="Time Offset") -> (x+y=w126:dbl)
    n31 = To Long Integer(number=w126) -> (32bit integer=w109:i32)
    "Elapsed Time" <- w109
    n32 = case shown="\"pulsed\"" w94 {
      tunnel: w146 -> [w224 w257 w289 w417 w440 w577 w667 w750 w802 w842 w883 w922 w957 w985 _ _ w1131 w1206 _ w1299 w1357 w1413 w1497 w1573 w1607]
      tunnel: w183 -> [w219 w253 w287 w424 w501 w585 w674 w758 w791 w831 w875 w915 w951 w978 w1011 w1067 w1109 w1188 w1233 w1286 w1344 w1401 w1491 w1569 w1609]
      tunnel: w182 -> [w218 w252 w278 w395 w486 w554 w643 w726 w792 w832 w876 w916 w952 w979 w1016 w1069 w1137 w1212 w1237 w1305 w1363 w1419 w1503 w1527 w1613]
      tunnel: w181 -> [w217 w251 w277 w394 w485 w553 w640 w723 w793 w833 w877 w917 w953 w980 w1015 w1040 w1136 w1211 w1236 w1304 w1362 w1418 w1502 w1526 w1612]
      tunnel: w180 -> [w216 w250 w286 w420 w461 w581 w670 w754 w801 w841 w874 w914 w950 w977 w1014 w1064 w1100 w1180 w1242 w1279 w1337 w1394 w1490 w1568 w1614]
      tunnel: w179 -> [w215 w249 w285 w422 w499 w583 w672 w756 w800 w840 w882 w921 w956 w984 w1013 w1049 w1135 w1210 w1245 w1303 w1361 w1417 w1501 w1577 w1615]
      tunnel: w178 -> [w214 w248 w284 w421 w498 w582 w671 w755 w799 w839 w881 w920 w955 w983 w1012 w1050 w1110 w1189 w1244 w1287 w1345 w1402 w1492 w1570 w1617]
      tunnel: [w218 w252 w276 w419 w496 w579 w669 w752 w792 w832 w876 w916 w952 w979 w1016 w1069 w1101 w1162 w1235 w1280 w1338 w1395 w1443 w1529 w1613] -> w177
      tunnel: [w217 w251 w275 w418 w495 w578 w668 w751 w793 w833 w877 w917 w953 w980 w1015 w1039 w1111 w1163 w1234 w1288 w1346 w1403 w1442 w1528 w1611] -> w108
      tunnel: [w216 w250 w286 w420 w457 w581 w670 w754 w794 w834 w874 w914 w950 w977 w1014 w1064 w1100 w1180 w1242 w1279 w1337 w1394 w1490 w1568 w1614] -> w176
      tunnel: [w215 w249 w285 w422 w499 w583 w672 w756 w800 w840 w882 w921 w956 w984 w1013 w1049 w1135 w1210 w1245 w1303 w1361 w1417 w1501 w1577 w1615] -> w175
      tunnel: [w214 w248 w284 w421 w498 w582 w671 w755 w799 w839 w881 w920 w955 w983 w1012 w1050 w1110 w1189 w1244 w1287 w1345 w1402 w1492 w1570 w1617] -> w174
      tunnel: [w219 w253 w287 w424 w501 w585 w674 w758 w791 w831 w875 w915 w951 w978 w1011 w1067 w1109 w1188 w1233 w1286 w1344 w1401 w1491 w1569 w1609] -> w57
      tunnel: w173 -> [_ _ _ w426 w505 w590 w677 w762 _ _ _ _ _ _ _ _ w1106 w1185 _ w1285 w1343 w1400 w1463 w1545 _]
      tunnel: "Gate" -> [_ _ _ w404 w489 w564 w654 w737 _ _ _ _ _ _ _ _ _ _ _ _ _ _ _ _ _]
      tunnel: "Drain 2" -> [_ _ _ w403 w488 w563 w653 w736 _ _ _ _ _ _ _ _ _ _ _ _ _ _ _ _ _]
      tunnel: "Panel Controls" -> [_ _ _ _ _ w562 w652 w735 _ _ _ _ _ _ _ _ _ _ _ _ _ _ _ _ _]
      tunnel: w169 -> [w213 w247 w283 w388 w479 w547 w638 w721 w798 w838 _ w913 w949 w976 w1010 w1051 w1096 w1176 w1238 w1275 w1333 w1390 w1486 w1564 w1618]
      tunnel: w168 -> [w212 w246 w282 w387 w478 w546 w637 w720 w797 w837 w880 _ w940 w982 w1009 w1052 w1097 w1177 w1239 w1276 w1334 w1391 w1487 w1565 w1619]
      tunnel: w167 -> [w211 w245 w281 w386 w477 w545 w636 w719 w796 w836 w879 w919 w954 _ w1008 w1053 w1098 w1178 w1240 w1277 w1335 w1392 w1488 w1566 w1620]
      tunnel: w166 -> [w210 w244 w280 w385 w476 w544 w639 w722 w795 w835 w878 w918 _ w981 w1007 w1054 w1099 w1179 w1241 w1278 w1336 w1393 w1489 w1567 w1621]
      tunnel: [w213 w247 w283 w388 w479 w547 w638 w721 w798 w838 w873 w913 w949 w976 w1010 w1051 w1096 w1176 w1238 w1275 w1333 w1390 w1486 w1564 w1618] -> w165
      tunnel: [w212 w246 w282 w387 w478 w546 w637 w720 w797 w837 w880 w905 w940 w982 w1009 w1052 w1097 w1177 w1239 w1276 w1334 w1391 w1487 w1565 w1619] -> w164
      tunnel: [w211 w245 w281 w386 w477 w545 w636 w719 w796 w836 w879 w919 w954 w975 w1008 w1053 w1098 w1178 w1240 w1277 w1335 w1392 w1488 w1566 w1620] -> w163
      tunnel: [w210 w244 w280 w385 w476 w544 w639 w722 w795 w835 w878 w918 w941 w981 w1007 w1054 w1099 w1179 w1241 w1278 w1336 w1393 w1489 w1567 w1621] -> w162
      tunnel: w161 -> [_ _ _ w380 w473 _ w632 _ _ _ _ _ _ _ _ _ _ _ _ _ _ _ _ _ _]
      tunnel: w160 -> [_ _ _ w378 w472 _ _ _ _ _ _ _ _ _ _ _ _ _ _ _ _ _ _ _ _]
      tunnel: [w209 w240 w273 w310 w449 w534 w629 w708 w790 w829 w872 w904 w939 w974 w1006 w1035 w1088 w1145 w1232 w1264 w1326 w1384 w1440 w1522 w1610] -> w72
      tunnel: w159 -> [w209 w240 w273 w375 w449 w534 w629 w708 w790 w829 w872 w904 w939 w974 w1006 w1035 w1088 w1145 w1232 w1264 w1326 w1384 w1440 w1522 w1610]
      tunnel: w126 -> [_ _ _ w372 w446 w532 w626 w705 _ _ _ _ _ _ _ w1033 w1086 w1158 _ w1261 w1323 w1381 w1437 w1518 _]
      tunnel: w157 -> [_ _ _ w369 w445 w530 w625 w704 _ _ _ _ _ _ _ w1031 w1084 w1157 _ w1260 w1322 w1380 w1436 w1519 _]
      tunnel: w109 -> [_ _ _ w364 _ _ _ _ _ _ _ _ _ _ _ _ _ _ _ _ _ _ _ _ _]
      tunnel: [w208 w239 w272 w318 w448 w533 w628 w707 w789 w828 w871 w903 w938 w973 w1005 w1034 w1087 w1160 w1231 w1263 w1325 w1383 w1439 w1521 w1616] -> w110
      tunnel: w155 -> [w208 w239 w272 w368 w448 w533 w628 w707 w789 w828 w871 w903 w938 w973 w1005 w1034 w1087 w1160 w1231 w1263 w1325 w1383 w1439 w1521 w1616]
      tunnel: [w207 w238 w271 w309 w444 w529 w624 w703 w788 w827 w870 w902 w937 w972 w1004 w1030 w1083 w1144 w1230 w1259 w1321 w1379 w1435 w1517 w1605] -> w71
      tunnel: w131 -> [w207 w238 w271 w362 w444 w529 w624 w703 w788 w827 w870 w902 w937 w972 w1004 w1030 w1083 w1144 w1230 w1259 w1321 w1379 w1435 w1517 w1605]
      tunnel: [w206 w237 w270 w355 w443 w528 w614 w702 w787 w826 w869 w901 w936 w971 w1003 w1029 w1082 w1156 w1229 w1258 w1320 w1378 w1434 w1516 w1604] -> w104
      tunnel: w117 -> [w206 w237 w270 w355 w443 w528 w614 w702 w787 w826 w869 w901 w936 w971 w1003 w1029 w1082 w1156 w1229 w1258 w1320 w1378 w1434 w1516 w1603]
      tunnel: [w205 w236 w269 w354 w442 w527 w613 w701 w786 w825 w868 w900 w935 w970 w1002 w1028 w1081 w1155 w1228 w1257 w1319 w1377 w1433 w1515 w1589] -> w112
      tunnel: w111 -> [w205 w236 w269 w354 w442 w527 w613 w701 w786 w825 w868 w900 w935 w970 w1002 w1028 w1081 w1155 w1228 w1257 w1319 w1377 w1433 w1515 w1589]
      tunnel: w109 -> [_ _ _ _ _ _ _ _ _ _ _ _ _ _ _ _ _ _ _ _ _ _ _ _ _]
      tunnel: [w204 w235 w268 w353 w441 w526 w612 w700 w785 w824 w867 w899 w934 w969 w1001 w1027 w1080 w1154 w1227 w1256 w1318 w1376 w1432 w1514 w1588] -> w105
      tunnel: w107 -> [w204 w235 w268 w353 w441 w526 w612 w700 w785 w824 w867 w899 w934 w969 w1001 w1027 w1080 w1154 w1227 w1256 w1318 w1376 w1432 w1514 w1588]
      tunnel: [w202 w233 w266 w303 w438 w524 w610 w698 w783 w823 w866 w897 w932 w967 w999 w1025 w1079 w1153 w1226 w1255 w1317 w1374 w1431 w1513 w1587] -> w65
      tunnel: w93 -> [w202 w233 w266 w349 w438 w524 w610 w698 w783 w823 w866 w897 w932 w967 w999 w1025 w1079 w1153 w1226 w1255 w1317 w1374 w1431 w1513 w1587]
      tunnel: [w203 w234 w267 w304 w439 w525 w611 w699 w784 w822 w865 w898 w933 w968 w1000 w1026 w1078 w1152 w1225 w1254 w1316 w1375 w1430 w1512 w1586] -> w66
      tunnel: w92 -> [w203 w234 w267 w348 w439 w525 w611 w699 w784 w822 w865 w898 w933 w968 w1000 w1026 w1078 w1152 w1225 w1254 w1316 w1375 w1430 w1512 w1586]
      tunnel: [w195 w226 w259 w308 w435 w522 w608 w696 w776 w820 w863 w895 w930 w965 w997 w1018 w1071 w1143 w1224 w1247 w1309 w1367 w1423 w1507 w1579] -> w70
      tunnel: w81 -> [w195 w226 w259 w338 w435 w522 w608 w696 w776 w820 w863 w895 w930 w965 w997 w1018 w1071 w1143 w1224 w1247 w1309 w1367 w1423 w1507 w1579]
      tunnel: [w194 w225 w258 w307 w436 w523 w609 w697 w775 w821 w864 w896 w931 w966 w998 w1017 w1070 w1142 w1223 w1246 w1308 w1366 w1422 w1506 w1578] -> w69
      tunnel: w80 -> [w194 w225 w258 w337 w436 w523 w609 w697 w775 w821 w864 w896 w931 w966 w998 w1017 w1070 w1142 w1223 w1246 w1308 w1366 w1422 w1506 w1578]
      tunnel: [w197 w228 w261 w313 w434 w520 w606 w694 w781 w818 w861 w893 w928 w963 w995 w1020 w1073 w1147 w1218 w1249 w1311 w1369 w1425 w1505 w1583] -> w63
      tunnel: w79 -> [w197 w228 w261 w334 w434 w520 w606 w694 w781 w818 w861 w893 w928 w963 w995 w1020 w1073 w1147 w1218 w1249 w1311 w1369 w1425 w1505 w1583]
      tunnel: [w196 w227 w260 w311 w437 w521 w607 w695 w782 w819 w862 w894 w929 w964 w996 w1019 w1072 w1146 w1217 w1248 w1310 w1368 w1424 w1504 w1582] -> w73
      tunnel: w78 -> [w196 w227 w260 w333 w437 w521 w607 w695 w782 w819 w862 w894 w929 w964 w996 w1019 w1072 w1146 w1217 w1248 w1310 w1368 w1424 w1504 w1582]
      tunnel: [w199 w230 w263 w302 w433 w518 w604 w692 w779 w816 w859 w891 w926 w961 w993 w1022 w1075 w1149 w1220 w1251 w1313 w1371 w1427 w1509 w1585] -> w64
      tunnel: w77 -> [w199 w230 w263 w330 w433 w518 w604 w692 w779 w816 w859 w891 w926 w961 w993 w1022 w1075 w1149 w1220 w1251 w1313 w1371 w1427 w1509 w1585]
      tunnel: [w198 w229 w262 w301 w432 w519 w605 w693 w780 w817 w860 w892 w927 w962 w994 w1021 w1074 w1148 w1219 w1250 w1312 w1370 w1426 w1508 w1584] -> w62
      tunnel: w76 -> [w198 w229 w262 w329 w432 w519 w605 w693 w780 w817 w860 w892 w927 w962 w994 w1021 w1074 w1148 w1219 w1250 w1312 w1370 w1426 w1508 w1584]
      tunnel: [w201 w232 w265 w306 w431 w516 w602 w690 w777 w814 w857 w889 w924 w959 w991 w1024 w1077 w1151 w1222 w1253 w1315 w1373 w1429 w1511 w1581] -> w68
      tunnel: w75 -> [w201 w232 w265 w326 w431 w516 w602 w690 w777 w814 w857 w889 w924 w959 w991 w1024 w1077 w1151 w1222 w1253 w1315 w1373 w1429 w1511 w1581]
      tunnel: [w200 w231 w264 w305 w430 w517 w603 w691 w778 w815 w858 w890 w925 w960 w992 w1023 w1076 w1150 w1221 w1252 w1314 w1372 w1428 w1510 w1580] -> w67
      tunnel: w74 -> [w200 w231 w264 w325 w430 w517 w603 w691 w778 w815 w858 w890 w925 w960 w992 w1023 w1076 w1150 w1221 w1252 w1314 w1372 w1428 w1510 w1580]
      frame "wait" {
        n33 = Index Array(array=w224, index=0 ("Index")) -> (element=w222:string)
        n34 = Decimal String To Number(string=w222, default (0L)=u32 0) -> (number=w221:u32)  [unwired: 1 in, 1 out]
        n35 = Wait (ms)(milliseconds to wait=w221) -> ()  [unwired: 1 out]
      }
      frame "wait-min" {
        n36 = Index Array(array=w257, index=0 ("Index")) -> (element=w255:string)
        n37 = Decimal String To Number(string=w255, default (0L)=u32 0) -> (number=w243:u32)  [unwired: 1 in, 1 out]
        n38 = Multiply(x=w243, y=u32 60000) -> (x*y=w242:u32)
        n39 = Wait (ms)(milliseconds to wait=w242) -> ()  [unwired: 1 out]
      }
      frame "standby" {
        n40 = Index Array(array=w289, index=0 ("Index")) -> (element=w279:string)
        n41 = case shown="\"off\", Default" w279 {
          tunnel: [":PAGE:SCON:STAN 0" ":PAGE:SCON:STAN 1"] -> w274
          frame "off", Default {
          }
          frame "on" {
          }
        }
        n42 = VISA Write(VISA resource name=w278, write buffer=w274, error in (no error)=w277) -> (VISA resource name out=w276:refnum<visa-resource-name>, error out=w275:errorcluster)  [unwired: 1 out]
      }
      frame "transfer" {
        # "Adjusts graph colors."
        # "Adjusts graph colors."
        # "Is off"
        # "Is on"
        # "Ion will be the middle element of the array. The calculation of the index is done only once, since Is, Id, and Ig have the same dimensions."
        # "Ig off"
        # "Ig on"
        # "Is min"
        # "Is max"
        # "Ig min"
        # "Ig max"
        # "abs(Ig)"
        # "abs(Is)"
        # "Id min"
        # "Id max"
        # "Y1: Is\nY2: Id\nY3: Ig"
        # "abs(Id)"
        # "Adjusts graph colors."
        # "Adjusts graph colors."
        # "Id off"
        # "Id on"
        # "Don't connect the error lines\nof the two Split blocks!"
        # "Adjusts graph colors."
        # "Time array"
        n43 = Delete From Array(array=w417, index=0 ("Index")) -> (deleted portion=w415:string, array with subset deleted=w414:string[])  [unwired: 1 in]
        n44 = Bundle By Name(cluster=w378, "Emergency Stop"=w426) -> (w379:T2)
        n45 = Number To Decimal String(number=w372) -> (decimal integer string=w371:string)  [unwired: 1 in]
        n46 = case shown="\"d\", Default" w415 {
          tunnel: [w428 w429] -> w413
          frame "s" {
            w428 = u16 0 items=["Single", "Double"] ("sweep mode")
          }
          frame "d", Default {
            w429 = u16 1 items=["Single", "Double"] ("sweep mode")
          }
        }
        n47 = Fract/Exp String To Number(string=w414) -> (number=w399:dbl[])  [unwired: 3 in, 1 out]
        n48 = Concatenate Strings(w424, "-transfer-" ("Prefix"), w371, w369, ".txt" ("Suffix (transfer)")) -> (w425:string)
        n49 = VISA Write(VISA resource name=w395, write buffer=":PAGE:CHAN:MODE SWE;" ("write buffer (\"\")"), error in (no error)=w394) -> (VISA resource name out=w392:refnum<visa-resource-name>, error out=w393:errorcluster)  [unwired: 1 out]
        n50 = String To Path(string=w425) -> (path=w423:path)
        n51 = Index Array(array=w399, index #1=0 ("Index")) -> (element #1=w412:dbl, element #2=w411:dbl, element #3=w410:dbl)  [unwired: 2 in]
        n52 = Delete From Array(array=w399, length=3 ("Length"), index=0 ("Index")) -> (array with subset deleted=w397:dbl[])  [unwired: 1 out]
        n53 = Build Array (concatenate)(w368, w364) -> (w318:i32[])
        n54 = Bundle By Name(cluster=w404, "Gate Start"=w412, "Gate Stop"=w411, "Gate Step (linear only)"=w410, "Gate Compliance"=w421, "Range mode"=w388, "Range"=w387) -> (w389:T4)
        n55 = control-ref of="Imax vs time"() -> (w347:refnum<vi>)
        n56 = control-ref of="Imin vs time"() -> (w346:refnum<vi>)
        n57 = control-ref of="Ion vs time"() -> (w315:refnum<vi>)
        n58 = control-ref of="Ioff vs time"() -> (w314:refnum<vi>)
        n59 = control-ref of="I vs Vg"() -> (w373:refnum<vi>)
        n60 = Index Array(array=w397, index #1=0 ("Index")) -> (element #1=w407:dbl, element #2=w406:dbl, element #3=w405:dbl)  [unwired: 2 in]
        n61 = call <vilib>:"compatOverwrite.vi"("overwrite (F)"=TRUE) -> ("overwrite?"=w377:T7)
        n62 = Bundle By Name(cluster=w403, "Drain Start"=w407, "Drain Stop"=w406, "Drain Step"=w405, "Drain Compliance"=w422, "Range mode"=w386, "Range"=w385) -> (w390:T5)
        n63 = call "4155C Transfer.vi"("VISA resource name in"=w392, "Gate"=w389, "Drain"=w390, "Timings"=w420, "error in (no error)"=w393, "SMU4"=w380, "sweep mode"=w413, "Panel Controls"=w379) -> ("VG"=w376:dbl[], "Outparams"=w384:T8, "VISA Resource Name out"=w419:refnum<visa-resource-name>, "IS"=w343:dbl[], "ID"=w345:dbl[], "IG"=w342:dbl[], "error out"=w365:errorcluster, "SMU4"=w381:dbl[])  [unwired: 12 in]
        n64 = Unbundle By Name(w384) -> ("V2 Step"=w383:dbl, "V2 Start"=w382:dbl, "Number of points"=w312:i32)
        n65 = Absolute Value(x=w343) -> (abs(x)=w328:dbl[])
        n66 = Absolute Value(x=w345) -> (abs(x)=w344:dbl[])
        n67 = Absolute Value(x=w342) -> (abs(x)=w331:dbl[])
        n68 = Array Size(array=w344) -> (size(s)=w352:i32)
        n69 = Divide(x=w352, y=2) -> (x/y=w295:dbl)
        n70 = Subtract(x=w295, y=1) -> (x-y=w294:dbl)
        n71 = Array Max & Min(array=w328) -> (max value=w335:dbl, min value=w336:dbl)  [unwired: 2 out]
        n72 = Array Max & Min(array=w344) -> (max value=w374:dbl, min value=w341:dbl)  [unwired: 2 out]
        n73 = Array Max & Min(array=w331) -> (max value=w340:dbl, min value=w339:dbl)  [unwired: 2 out]
        n74 = call "4155C Split array.vi"("Number of VAR2 steps"=w312, "Y2 data in"=w345, "X data in"=w376, "Y1 data in"=w343, "Y3 data in"=w342, "error in (no error)"=w365) -> ("Array of clusters"=w367:cluster{"Y data in":dbl[], "X data in":dbl[]}[], "error out"=w300:errorcluster)  [unwired: 1 in]
        n75 = Index Array(array=w328, index=w294) -> (element=w319:dbl)
        n76 = Index Array(array=w328, index=0) -> (element=w320:dbl)
        n77 = Index Array(array=w344, index=w294) -> (element=w321:dbl)
        n78 = Index Array(array=w344, index=0) -> (element=w322:dbl)
        n79 = Index Array(array=w331, index=w294) -> (element=w324:dbl)
        n80 = Index Array(array=w331, index=0) -> (element=w323:dbl)
        n81 = local write "Ig max"(w340) -> ()
        n82 = local write "Ig min"(w339) -> ()
        n83 = local write "Is max"(w335) -> ()
        n84 = local write "Is min"(w336) -> ()
        n85 = local write "Id max"(w374) -> ()
        n86 = local write "Id min"(w341) -> ()
        n87 = local write "I vs Vg"(w367) -> ()
        n88 = Build Array (concatenate)(w334, w335) -> (w313:dbl[])
        n89 = Build Array (concatenate)(w333, w336) -> (w311:dbl[])
        n90 = local write "Is off"(w320) -> ()
        n91 = local write "Is on"(w319) -> ()
        n92 = Build Array (concatenate)(w375, w374) -> (w310:dbl[])
        n93 = Build Array (concatenate)(w362, w341) -> (w309:dbl[])
        n94 = Build Array (concatenate)(w338, w340) -> (w308:dbl[])
        n95 = Build Array (concatenate)(w337, w339) -> (w307:dbl[])
        n96 = Build Array (concatenate)(w326, w319) -> (w306:dbl[])
        n97 = Build Array (concatenate)(w325, w320) -> (w305:dbl[])
        n98 = Build Array (concatenate)(w348, w321) -> (w304:dbl[])
        n99 = Build Array (concatenate)(w349, w322) -> (w303:dbl[])
        n100 = Build Array (concatenate)(w330, w324) -> (w302:dbl[])
        n101 = Build Array (concatenate)(w329, w323) -> (w301:dbl[])
        n102 = local write "Ig off"(w323) -> ()
        n103 = local write "Ig on"(w324) -> ()
        n104 = local write "Id off"(w322) -> ()
        n105 = local write "Id on"(w321) -> ()
        n106 = call "4155C Split array.vi"("Number of VAR2 steps"=w312, "Y2 data in"=w304, "X data in"=w318, "Y1 data in"=w306, "Y3 data in"=w302, "error in (no error)"=w300) -> ("Array of clusters"=w316:cluster{"Y data in":dbl[], "X data in":dbl[]}[], "error out"=w299:errorcluster)  [unwired: 1 in]
        n107 = call "4155C Split array.vi"("Number of VAR2 steps"=w312, "Y2 data in"=w303, "X data in"=w318, "Y1 data in"=w305, "Y3 data in"=w301, "error in (no error)"=w299) -> ("Array of clusters"=w317:cluster{"Y data in":dbl[], "X data in":dbl[]}[], "error out"=w298:errorcluster)  [unwired: 1 in]
        n108 = call "4155C Split array.vi"("Number of VAR2 steps"=w312, "Y2 data in"=w310, "X data in"=w318, "Y1 data in"=w313, "Y3 data in"=w308, "error in (no error)"=w298) -> ("Array of clusters"=w366:cluster{"Y data in":dbl[], "X data in":dbl[]}[], "error out"=w297:errorcluster)  [unwired: 1 in]
        n109 = call "4155C Split array.vi"("Number of VAR2 steps"=w312, "Y2 data in"=w309, "X data in"=w318, "Y1 data in"=w311, "Y3 data in"=w307, "error in (no error)"=w297) -> ("Array of clusters"=w363:cluster{"Y data in":dbl[], "X data in":dbl[]}[], "error out"=w296:errorcluster)  [unwired: 1 in]
        n110 = Open/Create/Replace File(file path (use dialog)=w423, error in=w296, operation (0:open)=w377) -> (refnum out=w360:refnum<file>, error out=w358:errorcluster)  [unwired: 3 in, 1 out]
        n111 = call "4155C Make Big 2d array.vi"("1D Var1"=w376, "1d IS"=w343, "1d ID"=w345, "1d IG"=w342, "1d SMU4"=w381, "SMU4"=w380, "VAR2 START"=w382, "Number of VAR2 steps"=w312, "VAR2 STEP"=w383, "VAR1 Name"="Vg", "Decimal places in header"=i8 1, "VAR2 Name"="Vd") -> ("Header array"=w361:string[], "Data array"=w359:dbl[][])  [unwired: 14 in]
        n112 = local write "Imax vs time"(w366) -> ()
        n113 = local write "Imin vs time"(w363) -> ()
        n114 = local write "Ion vs time"(w316) -> ()
        n115 = local write "Ioff vs time"(w317) -> ()
        n116 = call "4155C Config Chart Colours.vi"("Numeric"=w312, "XY Graph 2"=w347) -> ()  [unwired: 6 in]
        n117 = call "4155C Config Chart Colours.vi"("Numeric"=w312, "XY Graph 2"=w346) -> ()  [unwired: 6 in]
        n118 = call "4155C Config Chart Colours.vi"("Numeric"=w312, "XY Graph 2"=w315) -> ()  [unwired: 6 in]
        n119 = call "4155C Config Chart Colours.vi"("Numeric"=w312, "XY Graph 2"=w314) -> ()  [unwired: 6 in]
        n120 = call "4155C Config Chart Colours.vi"("Numeric"=w312, "XY Graph 2"=w373) -> ()  [unwired: 6 in]
        n121 = call "4155C Write array to file.vi"("Byte Stream File Refnum"=w360, "Header"=w361, "Data Array"=w359, "error in (no error)"=w358) -> ("dup refnum"=w357:refnum<file>, "error out"=w356:errorcluster)  [unwired: 1 in]
        n122 = Close File(refnum=w357, error in=w356) -> (error out=w418:errorcluster)  [unwired: 1 out]
      }
      frame "pulsedstressV" {
        w455 = 0
        n123 = Number To Decimal String(number=w446) -> (decimal integer string=w502:string)  [unwired: 1 in]
        n124 = Delete From Array(array=w440, index=0 ("Index")) -> (deleted portion=w493:string, array with subset deleted=w492:string[])  [unwired: 1 in]
        n125 = Bundle By Name(cluster=w472, "Emergency Stop"=w505) -> (w474:T2)
        n126 = VISA Write(VISA resource name=w486, write buffer=":PAGE:CHAN:MODE SWE;" ("write buffer (\"\")"), error in (no error)=w485) -> (VISA resource name out=w483:refnum<visa-resource-name>, error out=w484:errorcluster)  [unwired: 1 out]
        n127 = Concatenate Strings(w501, "-pulsedstressV-" ("Substring"), w502, w445, ".txt" ("Substring")) -> (w504:string)
        n128 = case shown="\"d\", Default" w493 {
          tunnel: [w514 w515] -> w491
          frame "s" {
            w514 = u16 0 items=["Single", "Double"] ("sweep mode")
          }
          frame "d", Default {
            w515 = u16 1 items=["Single", "Double"] ("sweep mode")
          }
        }
        n129 = Fract/Exp String To Number(string=w492) -> (number=w487:dbl[])  [unwired: 3 in, 1 out]
        n130 = String To Path(string=w504) -> (path=w500:path)
        n131 = Index Array(array=w487, index #1=0 ("Index")) -> (element #1=w464:dbl, element #2=w463:dbl, element #3=w460:dbl, element #4=w459:dbl, element #5=w458:dbl, element #6=w462:dbl)  [unwired: 5 in]
        n132 = Bundle By Name(cluster=w461, "Pulse period"=w459, "Base voltage"=w460, "Pulse width"=w458) -> (w457:T6)
        n133 = Unbundle By Name(w457) -> ("Pulse period"=w465:dbl)
        n134 = Bundle By Name(cluster=w489, "Gate Start"=w463, "Gate Stop"=w464, "Gate Step (linear only)"=0, "Gate Compliance"=w498, "Range mode"=w479, "Range"=w478) -> (w480:T4)
        n135 = call <vilib>:"compatOverwrite.vi"("overwrite (F)"=TRUE) -> ("overwrite?"=w450:T7)
        n136 = Bundle By Name(cluster=w488, "Drain Start"=w462, "Drain Stop"=w455, "Drain Step"=w455, "Drain Compliance"=w499, "Range mode"=w477, "Range"=w476) -> (w481:T5)
        n137 = call "4155C PulsedStressV.vi"("VISA resource name in"=w483, "sweep mode"=w491, "Panel Controls"=w474, "Gate"=w480, "Drain"=w481, "Timings"=w457, "error in (no error)"=w484, "SMU4"=w473) -> ("VISA Resource Name out"=w496:refnum<visa-resource-name>, "ID"=w453:dbl[], "IG"=w451:dbl[], "Outparams"=w475:T8, "error out"=w497:errorcluster)  [unwired: 3 in]
        n138 = Unbundle By Name(w475) -> ("Number of points"=w452:i32)  [unwired: 2 out]
        n139 = for {
          N: w452 -> [_]
          tunnel: [w511] -> w454 mode=indexing
          tunnel: w465 -> [w513]
          i -> [w512]
          n140 = Multiply(x=w513, y=w512) -> (x*y=w511:dbl)
        }
        n141 = Insert Into Array(array=dbl[][] [] ("Input Array"), new element=w454) -> (w466:dbl[][])  [unwired: 2 in]
        n142 = Insert Into Array(array=w466, new element=w453) -> (w471:dbl[][])  [unwired: 2 in]
        n143 = Insert Into Array(array=w471, new element=w451) -> (w470:dbl[][])  [unwired: 2 in]
        n144 = Transpose 2D Array(2D array=w470) -> (transposed array=w469:dbl[][])
        n145 = Open/Create/Replace File(file path (use dialog)=w500, error in=w497, operation (0:open)=w450) -> (refnum out=w508:refnum<file>, error out=w509:errorcluster)  [unwired: 3 in, 1 out]
        n146 = call "4155C Write array to file.vi"("Byte Stream File Refnum"=w508, "Header"=string[] ["Time /s", "Id /A", "Ig /A"], "Data Array"=w469, "error in (no error)"=w509) -> ("dup refnum"=w506:refnum<file>, "error out"=w507:errorcluster)  [unwired: 1 in]
        n147 = Close File(refnum=w506, error in=w507) -> (error out=w495:errorcluster)  [unwired: 1 out]
      }
      frame "transfer-fpp" {
        n148 = Number To Decimal String(number=w532) -> (decimal integer string=w586:string)  [unwired: 1 in]
        n149 = Bundle By Name(cluster=w562, "Emergency Stop"=w590) -> (w598:T1)
        n150 = Delete From Array(array=w577, index=0 ("Index")) -> (deleted portion=w575:string, array with subset deleted=w574:string[])  [unwired: 1 in]
        n151 = Concatenate Strings(w585, "-transferfpp-" ("Substring"), w586, w530, ".txt" ("Substring")) -> (w588:string)
        n152 = VISA Write(VISA resource name=w554, write buffer=":PAGE:CHAN:MODE SWE;" ("write buffer (\"\")"), error in (no error)=w553) -> (VISA resource name out=w551:refnum<visa-resource-name>, error out=w552:errorcluster)  [unwired: 1 out]
        n153 = case shown="\"d\", Default" w575 {
          tunnel: [w599 w600] -> w573
          frame "s" {
            w599 = u16 0 items=["Single", "Double"] ("sweep mode")
          }
          frame "d", Default {
            w600 = u16 1 items=["Single", "Double"] ("sweep mode")
          }
        }
        n154 = Fract/Exp String To Number(string=w574) -> (number=w558:dbl[])  [unwired: 3 in, 1 out]
        n155 = String To Path(string=w588) -> (path=w584:path)
        n156 = Index Array(array=w558, index #1=0 ("Index")) -> (element #1=w572:dbl, element #2=w571:dbl, element #3=w570:dbl)  [unwired: 2 in]
        n157 = Delete From Array(array=w558, length=3 ("Length"), index=0 ("Index")) -> (array with subset deleted=w556:dbl[])  [unwired: 1 out]
        n158 = Bundle By Name(cluster=w564, "Gate Start"=w572, "Gate Stop"=w571, "Gate Step (linear only)"=w570, "Gate Compliance"=w582, "Range mode"=w547, "Range"=w546) -> (w548:T4)
        n159 = Index Array(array=w556, index #1=0 ("Index")) -> (element #1=w567:dbl, element #2=w566:dbl, element #3=w565:dbl)  [unwired: 2 in]
        n160 = call <vilib>:"compatOverwrite.vi"("overwrite (F)"=TRUE) -> ("overwrite?"=w535:T7)
        n161 = Bundle By Name(cluster=w563, "Drain Start"=w567, "Drain Stop"=w566, "Drain Step"=w565, "Drain Compliance"=w583, "Range mode"=w545, "Range"=w544) -> (w549:T5)
        n162 = call "4155C Transfer-FPP.vi"("VISA resource name in"=w551, "Gate"=w548, "Drain"=w549, "Timings"=w581, "error in (no error)"=w552, "sweep mode"=w573, "Panel Controls"=w598) -> ("VG"=w589:dbl[], "Outparams"=w543:T8, "VISA Resource Name out"=w579:refnum<visa-resource-name>, "Vprobe2"=w539:dbl[], "ID"=w538:dbl[], "IG"=w537:dbl[], "Vprobe1"=w536:dbl[], "error out"=w580:errorcluster)  [unwired: 13 in]
        n163 = Unbundle By Name(w543) -> ("V2 Step"=w542:dbl, "V2 Start"=w541:dbl, "Number of points"=w540:i32)
        n164 = Open/Create/Replace File(file path (use dialog)=w584, error in=w580, operation (0:open)=w535) -> (refnum out=w595:refnum<file>, error out=w596:errorcluster)  [unwired: 3 in, 1 out]
        n165 = call "4155C Make Big 2d array FPP.vi"("1D Var1"=w589, "1d ID"=w538, "1d Vp2"=w539, "1d IG"=w537, "1d Vp1"=w536, "VAR2 START"=w541, "Number of VAR2 steps"=w540, "VAR2 STEP"=w542, "VAR1 Name"="Vg", "Decimal places in header"=i8 1, "VAR2 Name"="Vd") -> ("Header array"=w591:string[], "Data array"=w592:dbl[][])  [unwired: 15 in]
        n166 = call "4155C Write array to file.vi"("Byte Stream File Refnum"=w595, "Header"=w591, "Data Array"=w592, "error in (no error)"=w596) -> ("dup refnum"=w593:refnum<file>, "error out"=w594:errorcluster)  [unwired: 1 in]
        n167 = Close File(refnum=w593, error in=w594) -> (error out=w578:errorcluster)  [unwired: 1 out]
      }
      frame "output" {
        n168 = Number To Decimal String(number=w626) -> (decimal integer string=w675:string)  [unwired: 1 in]
        n169 = Bundle By Name(cluster=w652, "Emergency Stop"=w677) -> (w687:T1)
        n170 = Delete From Array(array=w667, index=0 ("Index")) -> (deleted portion=w665:string, array with subset deleted=w664:string[])  [unwired: 1 in]
        n171 = Concatenate Strings(w674, "-output-" ("Substring"), w675, w625, ".txt" ("Suffix (output)")) -> (w676:string)
        n172 = VISA Write(VISA resource name=w643, write buffer=":PAGE:CHAN:MODE SWE;" ("write buffer (\"\")"), error in (no error)=w640) -> (VISA resource name out=w642:refnum<visa-resource-name>, error out=w641:errorcluster)  [unwired: 1 out]
        n173 = case shown="\"d\", Default" w665 {
          tunnel: [w688 w689] -> w663
          frame "s" {
            w688 = u16 0 items=["Single", "Double"] ("sweep mode")
          }
          frame "d", Default {
            w689 = u16 1 items=["Single", "Double"] ("sweep mode")
          }
        }
        n174 = Fract/Exp String To Number(string=w664) -> (number=w646:dbl[])  [unwired: 3 in, 1 out]
        n175 = String To Path(string=w676) -> (path=w673:path)
        n176 = Index Array(array=w646, index #1=0 ("Index")) -> (element #1=w662:dbl, element #2=w661:dbl, element #3=w660:dbl)  [unwired: 2 in]
        n177 = Delete From Array(array=w646, length=3 ("Length"), index=0 ("Index")) -> (array with subset deleted=w645:dbl[])  [unwired: 1 out]
        n178 = control-ref of="I vs Vd"() -> (w616:refnum<vi>)
        n179 = Bundle By Name(cluster=w654, "Gate Start"=w662, "Gate Stop"=w661, "Gate Step (linear only)"=w660, "Gate Compliance"=w671, "Range mode"=w638, "Range"=w637) -> (w686:T4)
        n180 = Index Array(array=w645, index #1=0 ("Index")) -> (element #1=w657:dbl, element #2=w656:dbl, element #3=w655:dbl)  [unwired: 2 in]
        n181 = call <vilib>:"compatOverwrite.vi"("overwrite (F)"=TRUE) -> ("overwrite?"=w630:T7)
        n182 = Bundle By Name(cluster=w653, "Drain Start"=w657, "Drain Stop"=w656, "Drain Step"=w655, "Drain Compliance"=w672, "Range mode"=w636, "Range"=w639) -> (w685:T5)
        n183 = call "4155C Output.vi"("VISA resource name in"=w642, "Gate"=w686, "Drain"=w685, "Timings"=w670, "error in (no error)"=w641, "SMU4"=w632, "sweep mode"=w663, "Panel controls"=w687) -> ("VD"=w623:dbl[], "Outparams"=w634:T8, "VISA Resource Name out"=w669:refnum<visa-resource-name>, "IS"=w622:dbl[], "ID"=w621:dbl[], "IG"=w620:dbl[], "error out"=w618:errorcluster, "SMU4"=w631:dbl[])  [unwired: 12 in]
        n184 = Unbundle By Name(w634) -> ("V2 Step"=w635:dbl, "V2 Start"=w633:dbl, "Number of points"=w615:i32)
        n185 = call "4155C Split array.vi"("Number of VAR2 steps"=w615, "Y2 data in"=w621, "X data in"=w623, "Y1 data in"=w622, "Y3 data in"=w620, "error in (no error)"=w618) -> ("Array of clusters"=w619:cluster{"Y data in":dbl[], "X data in":dbl[]}[], "error out"=w617:errorcluster)  [unwired: 1 in]
        n186 = local write "I vs Vd"(w619) -> ()
        n187 = call "4155C Config Chart Colours.vi"("Numeric"=w615, "XY Graph 2"=w616) -> ()  [unwired: 6 in]
        n188 = Open/Create/Replace File(file path (use dialog)=w673, error in=w617, operation (0:open)=w630) -> (refnum out=w682:refnum<file>, error out=w683:errorcluster)  [unwired: 3 in, 1 out]
        n189 = call "4155C Make Big 2d array.vi"("1D Var1"=w623, "1d IS"=w622, "1d ID"=w621, "1d IG"=w620, "1d SMU4"=w631, "SMU4"=w632, "VAR2 START"=w633, "Number of VAR2 steps"=w615, "VAR2 STEP"=w635, "VAR1 Name"="Vd", "Decimal places in header"=i8 1, "VAR2 Name"="Vg") -> ("Header array"=w678:string[], "Data array"=w679:dbl[][])  [unwired: 14 in]
        n190 = call "4155C Write array to file.vi"("Byte Stream File Refnum"=w682, "Header"=w678, "Data Array"=w679, "error in (no error)"=w683) -> ("dup refnum"=w680:refnum<file>, "error out"=w681:errorcluster)  [unwired: 1 in]
        n191 = Close File(refnum=w680, error in=w681) -> (error out=w668:errorcluster)  [unwired: 1 out]
      }
      frame "output-fpp" {
        n192 = Number To Decimal String(number=w705) -> (decimal integer string=w759:string)  [unwired: 1 in]
        n193 = Bundle By Name(cluster=w735, "Emergency Stop"=w762) -> (w772:T1)
        n194 = Delete From Array(array=w750, index=0 ("Index")) -> (deleted portion=w748:string, array with subset deleted=w747:string[])  [unwired: 1 in]
        n195 = VISA Write(VISA resource name=w726, write buffer=":PAGE:CHAN:MODE SWE;" ("write buffer (\"\")"), error in (no error)=w723) -> (VISA resource name out=w725:refnum<visa-resource-name>, error out=w724:errorcluster)  [unwired: 1 out]
        n196 = Concatenate Strings(w758, "-outputfpp-" ("Substring"), w759, w704, ".txt" ("Substring")) -> (w761:string)
        n197 = case shown="\"d\", Default" w748 {
          tunnel: [w773 w774] -> w746
          frame "s" {
            w773 = u16 0 items=["Single", "Double"] ("sweep mode")
          }
          frame "d", Default {
            w774 = u16 1 items=["Single", "Double"] ("sweep mode")
          }
        }
        n198 = Fract/Exp String To Number(string=w747) -> (number=w729:dbl[])  [unwired: 3 in, 1 out]
        n199 = String To Path(string=w761) -> (path=w757:path)
        n200 = Index Array(array=w729, index #1=0 ("Index")) -> (element #1=w745:dbl, element #2=w744:dbl, element #3=w743:dbl)  [unwired: 2 in]
        n201 = Delete From Array(array=w729, length=3 ("Length"), index=0 ("Index")) -> (array with subset deleted=w728:dbl[])  [unwired: 1 out]
        n202 = Bundle By Name(cluster=w737, "Gate Start"=w745, "Gate Stop"=w744, "Gate Step (linear only)"=w743, "Gate Compliance"=w755, "Range mode"=w721, "Range"=w720) -> (w771:T4)
        n203 = Index Array(array=w728, index #1=0 ("Index")) -> (element #1=w740:dbl, element #2=w739:dbl, element #3=w738:dbl)  [unwired: 2 in]
        n204 = call <vilib>:"compatOverwrite.vi"("overwrite (F)"=TRUE) -> ("overwrite?"=w709:T7)
        n205 = Bundle By Name(cluster=w736, "Drain Start"=w740, "Drain Stop"=w739, "Drain Step"=w738, "Drain Compliance"=w756, "Range mode"=w719, "Range"=w722) -> (w770:T5)
        n206 = call "4155C Output-FPP.vi"("VISA resource name in"=w725, "Gate"=w771, "Drain"=w770, "Timings"=w754, "error in (no error)"=w724, "sweep mode"=w746, "Panel controls"=w772) -> ("VD"=w714:dbl[], "Outparams"=w717:T8, "VISA Resource Name out"=w752:refnum<visa-resource-name>, "Vprobe2"=w713:dbl[], "ID"=w712:dbl[], "IG"=w711:dbl[], "Vprobe1"=w710:dbl[], "error out"=w753:errorcluster)  [unwired: 13 in]
        n207 = Unbundle By Name(w717) -> ("V2 Step"=w718:dbl, "V2 Start"=w716:dbl, "Number of points"=w715:i32)
        n208 = Open/Create/Replace File(file path (use dialog)=w757, error in=w753, operation (0:open)=w709) -> (refnum out=w767:refnum<file>, error out=w768:errorcluster)  [unwired: 3 in, 1 out]
        n209 = call "4155C Make Big 2d array FPP.vi"("1D Var1"=w714, "1d ID"=w712, "1d Vp2"=w713, "1d IG"=w711, "1d Vp1"=w710, "VAR2 START"=w716, "Number of VAR2 steps"=w715, "VAR2 STEP"=w718, "VAR1 Name"="Vd", "Decimal places in header"=i8 1, "VAR2 Name"="Vg") -> ("Header array"=w763:string[], "Data array"=w764:dbl[][])  [unwired: 15 in]
        n210 = call "4155C Write array to file.vi"("Byte Stream File Refnum"=w767, "Header"=w763, "Data Array"=w764, "error in (no error)"=w768) -> ("dup refnum"=w765:refnum<file>, "error out"=w766:errorcluster)  [unwired: 1 in]
        n211 = Close File(refnum=w765, error in=w766) -> (error out=w751:errorcluster)  [unwired: 1 out]
      }
      frame "itime" {
        n212 = Delete From Array(array=w802, index=0 ("Index")) -> (deleted portion=w803:string)  [unwired: 1 in, 1 out]
        n213 = case shown="\"s\"" w803 {
          tunnel: w801 -> [w807 w809 w812]
          tunnel: [w806 w808 w811] -> w794
          frame "s" {
            w805 = u32 0 items=["short  ", "medium  ", "long  "] ("integration time 2")
            n214 = Bundle By Name(cluster=w807, "integration time"=w805) -> (w806:T6)
          }
          frame "m", Default {
            w810 = u32 1 items=["short  ", "medium  ", "long  "] ("integration time 2")
            n215 = Bundle By Name(cluster=w809, "integration time"=w810) -> (w808:T6)
          }
          frame "l" {
            w813 = u32 2 items=["short  ", "medium  ", "long  "] ("integration time 2")
            n216 = Bundle By Name(cluster=w812, "integration time"=w813) -> (w811:T6)
          }
        }
      }
      frame "pulsed" {
        n217 = Delete From Array(array=w842, index=0 ("Index")) -> (deleted portion=w843:string, array with subset deleted=w830:string[])  [unwired: 1 in]
        n218 = case shown="\"on\", Default" w843 {
          tunnel: w841 -> [w853 w856]
          tunnel: [w852 w855] -> w834
          tunnel: w830 -> [w850 _]
          frame "on", Default {
            w851 = u16 1 items=["Continuous", "Pulsed"] ("sweep method")
            n219 = Fract/Exp String To Number(string=w850) -> (number=w848:dbl[])  [unwired: 3 in, 1 out]
            n220 = Index Array(array=w848, index #1=0 ("Index")) -> (element #1=w847:dbl, element #2=w846:dbl, element #3=w845:dbl)  [unwired: 2 in]
            n221 = Bundle By Name(cluster=w853, "sweep method"=w851, "Pulse period"=w847, "Base voltage"=w846, "Pulse width"=w845) -> (w852:T6)
          }
          frame "off" {
            w854 = u16 0 items=["Continuous", "Pulsed"] ("sweep method")
            n222 = Bundle By Name(cluster=w856, "sweep method"=w854) -> (w855:T6)
          }
        }
      }
      frame "gaterangemode" {
        n223 = Delete From Array(array=w883, index=0 ("Index")) -> (deleted portion=w884:string)  [unwired: 1 in, 1 out]
        n224 = case shown="\"f\"" w884 {
          tunnel: [w886 w887 w888] -> w873
          frame "a", Default {
            w886 = u16 0 items=["Auto", "Limited", "Fixed"] ("Gate Range\nmode 2")
          }
          frame "f" {
            w887 = u16 2 items=["Auto", "Limited", "Fixed"] ("Gate Range\nmode 2")
          }
          frame "l" {
            w888 = u16 1 items=["Auto", "Limited", "Fixed"] ("Gate Range\nmode 2")
          }
        }
      }
      frame "gaterange" {
        (unwired) u8 11 items=["10fA  ", "100fA  ", "1nA  ", "10nA", "100nA", "1uA", "10uA", "100uA", "1mA", "10mA", "100mA", "1A"] ("Gate Range 2")
        n225 = Delete From Array(array=w922, index=0 ("Index")) -> (deleted portion=w912:string)  [unwired: 1 in, 1 out]
        n226 = Scan Value(string=w912, format string="") -> (value=w910:dbl)  [unwired: 1 in, 1 out]
        n227 = Logarithm Base 10(1:w910) -> (0:w909:dbl)
        n228 = Round To Nearest(number=w909) -> (nearest integer value=w908:dbl)
        n229 = Add(x=w908, y=11.0) -> (x+y=w906:dbl)
        n230 = To Unsigned Byte Integer(number=w906) -> (unsigned 8bit integer=w905:u8)
      }
      frame "drainrange" {
        (unwired) u8 11 items=["10fA  ", "100fA  ", "1nA  ", "10nA", "100nA", "1uA", "10uA", "100uA", "1mA", "10mA", "100mA", "1A"] ("Gate Range 2")
        n231 = Delete From Array(array=w957, index=0 ("Index")) -> (deleted portion=w948:string)  [unwired: 1 in, 1 out]
        n232 = Scan Value(string=w948, format string="") -> (value=w946:dbl)  [unwired: 1 in, 1 out]
        n233 = Logarithm Base 10(1:w946) -> (0:w945:dbl)
        n234 = Round To Nearest(number=w945) -> (nearest integer value=w944:dbl)
        n235 = Add(x=w944, y=11.0) -> (x+y=w942:dbl)
        n236 = To Unsigned Byte Integer(number=w942) -> (unsigned 8bit integer=w941:u8)
      }
      frame "drainrangemode" {
        n237 = Delete From Array(array=w985, index=0 ("Index")) -> (deleted portion=w986:string)  [unwired: 1 in, 1 out]
        n238 = case shown="\"f\"" w986 {
          tunnel: [w988 w989 w990] -> w975
          frame "a", Default {
            w988 = u16 0 items=["Auto", "Limited", "Fixed"] ("Gate Range\nmode 2")
          }
          frame "f" {
            w989 = u16 2 items=["Auto", "Limited", "Fixed"] ("Gate Range\nmode 2")
          }
          frame "l" {
            w990 = u16 1 items=["Auto", "Limited", "Fixed"] ("Gate Range\nmode 2")
          }
        }
      }
      frame "Error", Default {
      }
      frame "logfile" {
        n239 = Number To Decimal String(number=w1033) -> (decimal integer string=w1068:string)  [unwired: 1 in]
        n240 = Concatenate Strings(w1067, "logfile" ("Substring"), w1068, w1031, ".txt" ("Substring")) -> (w1065:string)
        n241 = String To Path(string=w1065) -> (path=w1038:path)
        n242 = Unbundle(w1064) -> ("integration time"=w1063:u32, "Short/Long integration time"=w1062:dbl, "hold time (sec)"=w1061:dbl, "delay time (sec)"=w1060:dbl, "Step Time (0 disables)"=w1059:dbl, "sweep method"=w1058:u16, "Pulse period"=w1057:dbl, "Base voltage"=w1056:dbl, "Pulse width"=w1055:dbl)
        n243 = Build Array(w1063, w1062, w1061, w1060, w1059, w1058, w1057, w1056, w1055, w1049, w1050, w1051, w1052, w1053, w1054) -> (w1042:dbl[])
        n244 = Insert Into Array(array=dbl[][] [] ("Input Array"), new element=w1042) -> (w1041:dbl[][])  [unwired: 2 in]
        n245 = call <vilib>:"compatOverwrite.vi"("overwrite (F)"=TRUE) -> ("overwrite?"=w1036:T7)
        n246 = Open/Create/Replace File(file path (use dialog)=w1038, error in=w1040, operation (0:open)=w1036) -> (refnum out=w1046:refnum<file>, error out=w1045:errorcluster)  [unwired: 3 in, 1 out]
        n247 = call "4155C Write array to file.vi"("Byte Stream File Refnum"=w1046, "Header"=string[] ["Int Time", "Short/Long Itime", "Hold time", "Delay time", "Step time", "Sweep method", "Pulse period", "Base Voltage", "Pulse width", "Drain compliance", "Gate compliance", "Gate range mode", "Gate range", "S/D range mode", "S/D range"], "Data Array"=w1041, "error in (no error)"=w1045) -> ("dup refnum"=w1048:refnum<file>, "error out"=w1047:errorcluster)  [unwired: 1 in]
        n248 = Close File(refnum=w1048, error in=w1047) -> (error out=w1039:errorcluster)  [unwired: 1 out]
      }
      frame "sample" {
        n249 = Number To Decimal String(number=w1086) -> (decimal integer string=w1134:string)  [unwired: 1 in]
        n250 = Fract/Exp String To Number(string=w1131) -> (number=w1092:dbl[])  [unwired: 3 in, 1 out]
        n251 = Concatenate Strings(w1109, "-sample-" ("Substring"), w1134, w1084, ".txt" ("Substring")) -> (w1132:string)
        n252 = Index Array(array=w1092, index=0 ("Index")) -> (element=w1129:dbl)
        n253 = String To Path(string=w1132) -> (path=w1113:path)
        n254 = Index Array(array=w1092, index=2 ("Index")) -> (element=w1125:dbl)
        n255 = Index Array(array=w1092, index=3 ("Index")) -> (element=w1094:dbl)
        n256 = Index Array(array=w1092, index=4 ("Index")) -> (element=w1091:dbl)
        n257 = call "4155C Config Sampling Measurements.vi"("Sampling interval"=w1091, "Sample time"=w1094, "Display on/off"=TRUE, "Timings"=w1100, "Num Points"=w1125, "error in (no error)"=w1136, "Drain Compliance"=w1135, "Gate Compliance"=w1110, "VISA session"=w1137) -> ("error out"=w1138:errorcluster, "dup VISA resource name"=w1139:refnum<visa-resource-name>)  [unwired: 1 in]
        n258 = Index Array(array=w1092, index=1 ("Index")) -> (element=w1126:dbl)
        n259 = call "4155C Take Sample.vi"("Emergency Stop"=w1106, "error in (no error)"=w1138, "Vd"=w1126, "Vg"=w1129, "VISA resource name in"=w1139) -> ("error out"=w1104:errorcluster, "Id"=w1141:dbl[], "Ig"=w1115:dbl[], "VISA Resource Name out"=w1102:refnum<visa-resource-name>, "Is"=w1140:dbl[], "Time"=w1119:dbl[])  [unwired: 1 in]
        n260 = Insert Into Array(array=dbl[][] [] ("Input Array"), new element=w1119) -> (w1118:dbl[][])  [unwired: 2 in]
        n261 = Insert Into Array(array=w1118, new element=w1115) -> (w1117:dbl[][])  [unwired: 2 in]
        n262 = Insert Into Array(array=w1117, new element=w1141) -> (w1116:dbl[][])  [unwired: 2 in]
        n263 = VISA Write(VISA resource name=w1102, write buffer=":DISP ON" ("write buffer (\"\")"), error in (no error)=w1104) -> (VISA resource name out=w1101:refnum<visa-resource-name>, error out=w1103:errorcluster)  [unwired: 1 out]
        n264 = Insert Into Array(array=w1116, new element=w1140) -> (w1108:dbl[][])  [unwired: 2 in]
        n265 = Transpose 2D Array(2D array=w1108) -> (transposed array=w1107:dbl[][])
        n266 = call <vilib>:"compatOverwrite.vi"("overwrite (F)"=TRUE) -> ("overwrite?"=w1089:T7)
        n267 = Open/Create/Replace File(file path (use dialog)=w1113, error in=w1103, operation (0:open)=w1089) -> (refnum out=w1122:refnum<file>, error out=w1121:errorcluster)  [unwired: 3 in, 1 out]
        n268 = call "4155C Write array to file.vi"("Byte Stream File Refnum"=w1122, "Header"=string[] ["Time /s", "Ig /A", "Id /A", "Is /A"], "Data Array"=w1107, "error in (no error)"=w1121) -> ("dup refnum"=w1124:refnum<file>, "error out"=w1123:errorcluster)  [unwired: 1 in]
        n269 = Close File(refnum=w1124, error in=w1123) -> (error out=w1111:errorcluster)  [unwired: 1 out]
      }
      frame "samplei" {
        n270 = Number To Decimal String(number=w1158) -> (decimal integer string=w1209:string)  [unwired: 1 in]
        n271 = Concatenate Strings(w1188, "-samplei-" ("Substring"), w1209, w1157, ".txt" ("Substring")) -> (w1207:string)
        n272 = Fract/Exp String To Number(string=w1206) -> (number=w1173:dbl[])  [unwired: 3 in, 1 out]
        n273 = String To Path(string=w1207) -> (path=w1191:path)
        n274 = Index Array(array=w1173, index=4 ("Index")) -> (element=w1167:dbl)
        n275 = Index Array(array=w1173, index=3 ("Index")) -> (element=w1168:dbl)
        n276 = Index Array(array=w1173, index=1 ("Index")) -> (element=w1170:dbl)
        n277 = Index Array(array=w1173, index=0 ("Index")) -> (element=w1171:dbl)
        n278 = Index Array(array=w1173, index=2 ("Index")) -> (element=w1169:dbl)
        n279 = call "4155C Config SamplingI Measurements.vi"("Sample time"=w1169, "Display on/off"=TRUE, "Timings"=w1180, "Num Points"=w1170, "error in (no error)"=w1211, "Sampling interval"=w1168, "VISA session"=w1212) -> ("error out"=w1213:errorcluster, "dup VISA resource name"=w1214:refnum<visa-resource-name>)  [unwired: 3 in]
        n280 = call "4155C Take SampleI.vi"("Emergency Stop"=w1185, "error in (no error)"=w1213, "Idg 2"=w1171, "Vdg compliance 2"=w1167, "VISA resource name in"=w1214) -> ("error out"=w1183:errorcluster, "Idg"=w1216:dbl[], "Vdg"=w1193:dbl[], "VISA Resource Name out"=w1181:refnum<visa-resource-name>, "Is"=w1215:dbl[], "Time"=w1197:dbl[])  [unwired: 1 in]
        n281 = Insert Into Array(array=dbl[][] [] ("Input Array"), new element=w1197) -> (w1196:dbl[][])  [unwired: 2 in]
        n282 = Insert Into Array(array=w1196, new element=w1193) -> (w1195:dbl[][])  [unwired: 2 in]
        n283 = Insert Into Array(array=w1195, new element=w1216) -> (w1194:dbl[][])  [unwired: 2 in]
        n284 = VISA Write(VISA resource name=w1181, write buffer=":DISP ON" ("write buffer (\"\")"), error in (no error)=w1183) -> (VISA resource name out=w1166:refnum<visa-resource-name>, error out=w1182:errorcluster)  [unwired: 1 out]
        n285 = Insert Into Array(array=w1194, new element=w1215) -> (w1187:dbl[][])  [unwired: 2 in]
        n286 = call <vilib>:"compatOverwrite.vi"("overwrite (F)"=TRUE) -> ("overwrite?"=w1161:T7)
        n287 = Open/Create/Replace File(file path (use dialog)=w1191, error in=w1182, operation (0:open)=w1161) -> (refnum out=w1200:refnum<file>, error out=w1199:errorcluster)  [unwired: 3 in, 1 out]
        n288 = Transpose 2D Array(2D array=w1187) -> (transposed array=w1186:dbl[][])
        n289 = call "4155C Write array to file.vi"("Byte Stream File Refnum"=w1200, "Header"=string[] ["Time /s", "Vdg /V", "Idg /A", "Is /A"], "Data Array"=w1186, "error in (no error)"=w1199) -> ("dup refnum"=w1202:refnum<file>, "error out"=w1201:errorcluster)  [unwired: 1 in]
        n290 = Close File(refnum=w1202, error in=w1201) -> (error out=w1164:errorcluster)  [unwired: 1 out]
        n291 = VISA Write(VISA resource name=w1166, write buffer=";:PAGE:SCON:STAN OFF;:PAGE:CHAN:VSU2:DIS;" ("write buffer (\"\")"), error in (no error)=w1164) -> (VISA resource name out=w1162:refnum<visa-resource-name>, error out=w1163:errorcluster)  [unwired: 1 out]
      }
      frame "#" {
        n292 = VISA Write(VISA resource name=w1237, write buffer=":DISP ON" ("write buffer (\"\")"), error in (no error)=w1236) -> (VISA resource name out=w1235:refnum<visa-resource-name>, error out=w1234:errorcluster)  [unwired: 1 out]
      }
      frame "stressV" {
        n293 = Number To Decimal String(number=w1261) -> (decimal integer string=w1302:string)  [unwired: 1 in]
        n294 = Concatenate Strings(w1286, "-stressV-" ("Substring"), w1302, w1260, ".txt" ("Substring")) -> (w1300:string)
        n295 = Fract/Exp String To Number(string=w1299) -> (number=w1272:dbl[])  [unwired: 3 in, 1 out]
        n296 = String To Path(string=w1300) -> (path=w1290:path)
        n297 = Index Array(array=w1272, index=3 ("Index")) -> (element=w1269:dbl)
        n298 = Index Array(array=w1272, index=1 ("Index")) -> (element=w1267:dbl)
        n299 = Index Array(array=w1272, index=0 ("Index")) -> (element=w1266:dbl)
        n300 = Index Array(array=w1272, index=4 ("Index")) -> (element=w1271:dbl)
        n301 = Index Array(array=w1272, index=2 ("Index")) -> (element=w1268:dbl)
        n302 = call "4155C Config V Stress.vi"("VISA session"=w1305, "ID compliance"=w1269, "VD"=w1267, "VG"=w1266, "IG compliance"=w1268, "error in (no error)"=w1304, "Display on/off"=TRUE) -> ("dup VISA resource name"=w1307:refnum<visa-resource-name>, "error out"=w1306:errorcluster)
        n303 = call "4155C Apply Stress.vi"("error in (no error)"=w1306, "Duration"=w1271, "Emergency Stop"=w1285, "VISA resource name in"=w1307) -> ("error out"=w1283:errorcluster, "VISA Resource Name out"=w1281:refnum<visa-resource-name>)
        n304 = VISA Write(VISA resource name=w1281, write buffer=":DISP ON" ("write buffer (\"\")"), error in (no error)=w1283) -> (VISA resource name out=w1280:refnum<visa-resource-name>, error out=w1282:errorcluster)  [unwired: 1 out]
        n305 = call <vilib>:"compatOverwrite.vi"("overwrite (F)"=TRUE) -> ("overwrite?"=w1265:T7)
        n306 = Open/Create/Replace File(file path (use dialog)=w1290, error in=w1282, operation (0:open)=w1265) -> (refnum out=w1293:refnum<file>, error out=w1292:errorcluster)  [unwired: 3 in, 1 out]
        n307 = call "4155C Write array to file.vi"("Byte Stream File Refnum"=w1293, "Header"=string[] ["V stress completed successfully", ""], "error in (no error)"=w1292) -> ("dup refnum"=w1295:refnum<file>, "error out"=w1294:errorcluster)  [unwired: 2 in]
        n308 = Close File(refnum=w1295, error in=w1294) -> (error out=w1288:errorcluster)  [unwired: 1 out]
      }
      frame "stressI" {
        n309 = Number To Decimal String(number=w1323) -> (decimal integer string=w1360:string)  [unwired: 1 in]
        n310 = Concatenate Strings(w1344, "-stressI-" ("Substring"), w1360, w1322, ".txt" ("Substring")) -> (w1358:string)
        n311 = Fract/Exp String To Number(string=w1357) -> (number=w1332:dbl[])  [unwired: 3 in, 1 out]
        n312 = Index Array(array=w1332, index=1 ("Index")) -> (element=w1328:dbl)
        n313 = Index Array(array=w1332, index=0 ("Index")) -> (element=w1329:dbl)
        n314 = call "4155C Config I Stress.vi"("VISA session"=w1363, "IDG"=w1329, "VDG compliance"=w1328, "error in (no error)"=w1362, "Display on/off"=TRUE) -> ("dup VISA resource name"=w1365:refnum<visa-resource-name>, "error out"=w1364:errorcluster)
        n315 = Index Array(array=w1332, index=2 ("Index")) -> (element=w1330:dbl)
        n316 = String To Path(string=w1358) -> (path=w1348:path)
        n317 = call "4155C Apply Stress.vi"("error in (no error)"=w1364, "Duration"=w1330, "Emergency Stop"=w1343, "VISA resource name in"=w1365) -> ("error out"=w1341:errorcluster, "VISA Resource Name out"=w1339:refnum<visa-resource-name>)
        n318 = VISA Write(VISA resource name=w1339, write buffer=":DISP ON" ("write buffer (\"\")"), error in (no error)=w1341) -> (VISA resource name out=w1338:refnum<visa-resource-name>, error out=w1340:errorcluster)  [unwired: 1 out]
        n319 = call <vilib>:"compatOverwrite.vi"("overwrite (F)"=TRUE) -> ("overwrite?"=w1327:T7)
        n320 = Open/Create/Replace File(file path (use dialog)=w1348, error in=w1340, operation (0:open)=w1327) -> (refnum out=w1351:refnum<file>, error out=w1350:errorcluster)  [unwired: 3 in, 1 out]
        n321 = call "4155C Write array to file.vi"("Byte Stream File Refnum"=w1351, "Header"=string[] ["I stress completed successfully", ""], "error in (no error)"=w1350) -> ("dup refnum"=w1353:refnum<file>, "error out"=w1352:errorcluster)  [unwired: 2 in]
        n322 = Close File(refnum=w1353, error in=w1352) -> (error out=w1346:errorcluster)  [unwired: 1 out]
      }
      frame "vsu2pulse" {
        n323 = Number To Decimal String(number=w1381) -> (decimal integer string=w1416:string)  [unwired: 1 in]
        n324 = Concatenate Strings(w1401, "-vsu2-" ("Substring"), w1416, w1380, ".txt" ("Substring")) -> (w1414:string)
        n325 = Fract/Exp String To Number(string=w1413) -> (number=w1389:dbl[])  [unwired: 3 in, 1 out]
        n326 = String To Path(string=w1414) -> (path=w1405:path)
        n327 = Index Array(array=w1389, index=1 ("Index")) -> (element=w1388:dbl)
        n328 = Index Array(array=w1389, index=0 ("Index")) -> (element=w1386:dbl)
        n329 = call "4155C Config VSU2 Stress.vi"("error in (no error)"=w1418, "VSU2"=w1386, "Display on/off"=TRUE, "VISA session"=w1419) -> ("error out"=w1420:errorcluster, "dup VISA resource name"=w1421:refnum<visa-resource-name>)
        n330 = call "4155C Apply Stress.vi"("error in (no error)"=w1420, "Duration"=w1388, "Emergency Stop"=w1400, "VISA resource name in"=w1421) -> ("error out"=w1398:errorcluster, "VISA Resource Name out"=w1396:refnum<visa-resource-name>)
        n331 = VISA Write(VISA resource name=w1396, write buffer=":DISP ON" ("write buffer (\"\")"), error in (no error)=w1398) -> (VISA resource name out=w1395:refnum<visa-resource-name>, error out=w1397:errorcluster)  [unwired: 1 out]
        n332 = call <vilib>:"compatOverwrite.vi"("overwrite (F)"=TRUE) -> ("overwrite?"=w1385:T7)
        n333 = Open/Create/Replace File(file path (use dialog)=w1405, error in=w1397, operation (0:open)=w1385) -> (refnum out=w1408:refnum<file>, error out=w1407:errorcluster)  [unwired: 3 in, 1 out]
        n334 = call "4155C Write array to file.vi"("Byte Stream File Refnum"=w1408, "Header"=string[] ["VSU2 pulse completed successfully", ""], "error in (no error)"=w1407) -> ("dup refnum"=w1410:refnum<file>, "error out"=w1409:errorcluster)  [unwired: 2 in]
        n335 = Close File(refnum=w1410, error in=w1409) -> (error out=w1403:errorcluster)  [unwired: 1 out]
      }
      frame "sample-fpp" {
        w1448 = string[] ["Time /s", "Id VgVd /A", "Ig VgVd /A", "Vp1 VgVd /V", "Vp2 VgVd /V"] ("Header")
        w1452 = "%d" ("format string")
        n336 = Number To Decimal String(number=w1437) -> (decimal integer string=w1500:string)  [unwired: 1 in]
        n337 = Fract/Exp String To Number(string=w1497) -> (number=w1485:dbl[])  [unwired: 3 in, 1 out]
        n338 = Concatenate Strings(w1491, "-samplefpp-" ("Substring"), w1500, w1436, ".txt" ("Substring")) -> (w1498:string)
        n339 = String To Path(string=w1498) -> (path=w1460:path)
        n340 = Index Array(array=w1485, index=0 ("Index")) -> (element=w1446:dbl)
        n341 = Index Array(array=w1485, index=1 ("Index")) -> (element=w1445:dbl)
        n342 = Index Array(array=w1485, index=2 ("Index")) -> (element=w1493:dbl)
        n343 = Index Array(array=w1485, index=3 ("Index")) -> (element=w1483:dbl)
        n344 = call "4155C Config Sampling Measurements FPP.vi"("VISA session"=w1503, "Num Points"=w1493, "Vg"=w1446, "Display on/off"=TRUE, "Gate Compliance"=w1492, "Drain Compliance"=w1501, "Standby"="Standby", "error in (no error)"=w1502, "Timings"=w1490, "Vd"=w1445, "Sample time"=w1483) -> ("dup VISA resource name"=w1462:refnum<visa-resource-name>, "error out"=w1461:errorcluster)  [unwired: 3 in]
        n345 = Number To Decimal String(number=w1446) -> (decimal integer string=w1472:string)  [unwired: 1 in]
        n346 = call "4155C Take Sample FPP.vi"("VISA resource name in"=w1462, "error in (no error)"=w1461, "Emergency Stop"=w1463) -> ("Time"=w1467:dbl[], "Vp1"=w1477:dbl[], "VISA Resource Name out"=w1443:refnum<visa-resource-name>, "Ig"=w1465:dbl[], "Id"=w1466:dbl[], "Vp2"=w1475:dbl[], "error out"=w1464:errorcluster)  [unwired: 10 in]
        n347 = Insert Into Array(array=dbl[][] [] ("Input Array"), new element=w1467) -> (w1481:dbl[][])  [unwired: 2 in]
        n348 = Number To Decimal String(number=w1445) -> (decimal integer string=w1470:string)  [unwired: 1 in]
        n349 = Insert Into Array(array=w1481, new element=w1466) -> (w1480:dbl[][])  [unwired: 2 in]
        n350 = Concatenate Strings("(Vg = " ("Substring"), w1472, "V, Vd = " ("Substring"), w1470, "V)" ("Substring")) -> (w1468:string)
        n351 = Insert Into Array(array=w1480, new element=w1465) -> (w1479:dbl[][])  [unwired: 2 in]
        n352 = Insert Into Array(array=w1479, new element=w1477) -> (w1476:dbl[][])  [unwired: 2 in]
        n353 = Insert Into Array(array=w1476, new element=w1475) -> (w1444:dbl[][])  [unwired: 2 in]
        n354 = Transpose 2D Array(2D array=w1444) -> (transposed array=w1474:dbl[][])
        n355 = call <vilib>:"compatOverwrite.vi"("overwrite (F)"=TRUE) -> ("overwrite?"=w1441:T7)
        n356 = Open/Create/Replace File(file path (use dialog)=w1460, error in=w1464, operation (0:open)=w1441) -> (refnum out=w1457:refnum<file>, error out=w1458:errorcluster)  [unwired: 3 in, 1 out]
        n357 = Array To Spreadsheet String(array=w1448, 3:w1452) -> (spreadsheet string=w1454:string)  [unwired: 1 in]
        n358 = Search and Replace String(replace all?=TRUE ("replace all? (F)"), input string=w1454, search string="VgVd", replace string=w1468) -> (result string=w1450:string)  [unwired: 4 in, 3 out]
        n359 = Spreadsheet String To Array(format string=w1452, spreadsheet string=w1450, array type (2D Dbl)=w1448) -> (array=w1449:string[])  [unwired: 1 in]
        n360 = call "4155C Write array to file.vi"("Byte Stream File Refnum"=w1457, "Header"=w1449, "Data Array"=w1474, "error in (no error)"=w1458) -> ("dup refnum"=w1455:refnum<file>, "error out"=w1456:errorcluster)  [unwired: 1 in]
        n361 = Close File(refnum=w1455, error in=w1456) -> (error out=w1442:errorcluster)  [unwired: 1 out]
      }
      frame "resample-fpp" {
        w1532 = string[] ["Time /s", "Id VgVd /A", "Ig VgVd /A", "Vp1 VgVd /V", "Vp2 VgVd /V"] ("Header")
        w1536 = "%d" ("format string")
        n362 = Number To Decimal String(number=w1518) -> (decimal integer string=w1576:string)  [unwired: 1 in]
        n363 = Fract/Exp String To Number(string=w1573) -> (number=w1525:dbl[])  [unwired: 3 in, 1 out]
        n364 = Concatenate Strings(w1569, "-resamplefpp-" ("Substring"), w1576, w1519, ".txt" ("Substring")) -> (w1574:string)
        n365 = String To Path(string=w1574) -> (path=w1544:path)
        n366 = Index Array(array=w1525, index=0 ("Index")) -> (element=w1531:dbl)
        n367 = Index Array(array=w1525, index=1 ("Index")) -> (element=w1530:dbl)
        n368 = Number To Decimal String(number=w1531) -> (decimal integer string=w1554:string)  [unwired: 1 in]
        n369 = call "4155C Take Sample FPP.vi"("VISA resource name in"=w1527, "error in (no error)"=w1526, "Emergency Stop"=w1545) -> ("Time"=w1549:dbl[], "Vp1"=w1559:dbl[], "VISA Resource Name out"=w1529:refnum<visa-resource-name>, "Ig"=w1547:dbl[], "Id"=w1548:dbl[], "Vp2"=w1557:dbl[], "error out"=w1546:errorcluster)  [unwired: 10 in]
        n370 = Insert Into Array(array=dbl[][] [] ("Input Array"), new element=w1549) -> (w1563:dbl[][])  [unwired: 2 in]
        n371 = Number To Decimal String(number=w1530) -> (decimal integer string=w1552:string)  [unwired: 1 in]
        n372 = Insert Into Array(array=w1563, new element=w1548) -> (w1562:dbl[][])  [unwired: 2 in]
        n373 = Concatenate Strings("(Vg = " ("Substring"), w1554, "V, Vd = " ("Substring"), w1552, "V)" ("Substring")) -> (w1550:string)
        n374 = Insert Into Array(array=w1562, new element=w1547) -> (w1561:dbl[][])  [unwired: 2 in]
        n375 = Insert Into Array(array=w1561, new element=w1559) -> (w1558:dbl[][])  [unwired: 2 in]
        n376 = Insert Into Array(array=w1558, new element=w1557) -> (w1524:dbl[][])  [unwired: 2 in]
        n377 = call <vilib>:"compatOverwrite.vi"("overwrite (F)"=TRUE) -> ("overwrite?"=w1523:T7)
        n378 = Open/Create/Replace File(file path (use dialog)=w1544, error in=w1546, operation (0:open)=w1523) -> (refnum out=w1541:refnum<file>, error out=w1542:errorcluster)  [unwired: 3 in, 1 out]
        n379 = Array To Spreadsheet String(array=w1532, 3:w1536) -> (spreadsheet string=w1538:string)  [unwired: 1 in]
        n380 = Transpose 2D Array(2D array=w1524) -> (transposed array=w1556:dbl[][])
        n381 = Search and Replace String(replace all?=TRUE ("replace all? (F)"), input string=w1538, search string="VgVd", replace string=w1550) -> (result string=w1534:string)  [unwired: 4 in, 3 out]
        n382 = Spreadsheet String To Array(format string=w1536, spreadsheet string=w1534, array type (2D Dbl)=w1532) -> (array=w1533:string[])  [unwired: 1 in]
        n383 = call "4155C Write array to file.vi"("Byte Stream File Refnum"=w1541, "Header"=w1533, "Data Array"=w1556, "error in (no error)"=w1542) -> ("dup refnum"=w1539:refnum<file>, "error out"=w1540:errorcluster)  [unwired: 1 in]
        n384 = Close File(refnum=w1539, error in=w1540) -> (error out=w1528:errorcluster)  [unwired: 1 out]
      }
      frame "serial" {
        n385 = local read "Termination char\n(0xA = '\\n' = LF)\n(0xD = '\\r' = CR)"() -> (w1599:u8)
        n386 = local read "Enable Termination\nChar (T)"() -> (w1600:bool)
        n387 = Index Array(array=w1607, index=0 ("Index")) -> (element=w1606:string)
        n388 = local read "parity"() -> (w1590:u16)
        n389 = local read "Delay before read (ms)"() -> (w1601:u32)
        n390 = local read "byte count"() -> (w1598:u32)
        n391 = local read "Timeout (ms)"() -> (w1597:u32)
        n392 = local read "VISA resource name"() -> (w1594:refnum<visa-resource-name>)
        n393 = local read "baud rate"() -> (w1593:u32)
        n394 = local read "Serial End Mode for Reads"() -> (w1592:u16)
        n395 = local read "data bits"() -> (w1591:u16)
        n396 = local read "stop bits"() -> (w1596:u16)
        n397 = local read "flow control"() -> (w1595:u16)
        n398 = call "Serial write and read v0.5.vi"("Delay before read (ms)"=w1601, "Termination char\n(0xA = '\\n' = LF)\n(0xD = '\\r' = CR)"=w1599, "Enable Termination\nChar (T)"=w1600, "parity"=w1590, "stop bits"=w1596, "string to write"=w1606, "flow control"=w1595, "byte count"=w1598, "Serial Settings:Serial End Mode for Reads"=w1592, "Timeout (ms)"=w1597, "error in (no error)"=w1612, "VISA resource name"=w1594, "baud rate"=w1593, "data bits"=w1591) -> ("Serial port output"=w1602:string, "error out"=w1611:errorcluster)
        n399 = Build Array (concatenate)(w1602, w1603) -> (w1604:string[])
      }
    }
    n400 = Build Array(w110, w63, w73, w72, w71, w70, w69, w68, w67, w66, w65, w64, w62) -> (w134:dbl[][])
    n401 = Transpose 2D Array(2D array=w134) -> (transposed array=w133:dbl[][])
    n402 = Concatenate Strings(w57, "Imax_Imin_Ion_Ioff_vs_time.txt" ("Suffix (Imax,Imin,Ion,Ioff)")) -> (w144:string)
    n403 = Build Array(w95, "Is max (A)" ("VAR2 Name"), "Is min (A)" ("VAR2 Name"), "Id max (A)" ("VAR2 Name"), "Id min (A)" ("VAR2 Name"), "Ig max (A)" ("VAR2 Name"), "Ig min (A)" ("VAR2 Name"), "Is on (A)" ("VAR2 Name"), "Is off (A)" ("VAR2 Name"), "Id on (A)" ("VAR2 Name"), "Id off (A)" ("VAR2 Name"), "Ig on (A)" ("VAR2 Name"), "Ig off (A)" ("VAR2 Name")) -> (w139:string[])
    n404 = Array To Spreadsheet String(array=w133, 3:"%e" ("format string")) -> (spreadsheet string=w137:string)  [unwired: 1 in]
    n405 = Array To Spreadsheet String(array=w139, 3:"" ("format string")) -> (spreadsheet string=w138:string)  [unwired: 1 in]
    n406 = String To Path(string=w144) -> (path=w143:path)
    n407 = Build Array(w138, w137) -> (w136:string[])
    n408 = Write to Text File(file (use dialog)=w143, text=w136, error in=w108) -> (refnum out=w145:refnum<file>, error out=w135:errorcluster)  [unwired: 1 in, 1 out]
    n409 = Close File(refnum=w145, error in=w135) -> (error out=w60:errorcluster)  [unwired: 1 out]
    n410 = Concatenate Strings(w57, "serial_port_output.txt" ("Suffix (serial port log)")) -> (w114:string)
    n411 = String To Path(string=w114) -> (path=w113:path)
    n412 = Build Array(w95, "Serial port input" ("VAR2 Name"), "Pump status" ("VAR2 Name"), "Serial port output: ") -> (w99:string[])
    n413 = Array To Spreadsheet String(array=w105, 3:"" ("format string")) -> (spreadsheet string=w96:string)  [unwired: 1 in]
    n414 = Array To Spreadsheet String(array=w99, 3:"" ("format string")) -> (spreadsheet string=w97:string)  [unwired: 1 in]
    n415 = Build Array(w97, w96) -> (w98:string[])
    n416 = Array To Spreadsheet String(array=w104, 3:"" ("format string")) -> (spreadsheet string=w119:string)  [unwired: 1 in]
    n417 = Write to Text File(file (use dialog)=w113, text=w98, error in=w60) -> (refnum out=w115:refnum<file>, error out=w116:errorcluster)  [unwired: 1 in, 1 out]
    n418 = Close File(refnum=w115, error in=w116) -> (error out=w59:errorcluster)  [unwired: 1 out]
    n419 = local write "Serial port data"(w119) -> ()
  }
  "error out" <- w16
